vi "reporter2.vi"(1 "file path (dialog if empty)":path=path "C:/Users/Dimitris/Desktop/16_1_15.xls") -> (0 "output array 2":string[][](array[string]))   [LabVIEW 2012]
uses:
  <vilib>/Utility/file.llb/Write To Spreadsheet File (string).vi
  <vilib>/Utility/file.llb/Read From Spreadsheet File (DBL).vi
panel:
  out "output array 4":string[][](array[string])
  out "radiation_array 3":dbl[](array[numeric])
  out "radiation_array 2":dbl[](array[numeric])
  out "Panel7 acc":dbl[](array[numeric])
  out "Panel7 array":dbl[](array[numeric])
  out "Panel 6 acc":dbl[](array[numeric])
  out "Panel 6 array":dbl[](array[numeric])
  out "Panel 5 acc":dbl[](array[numeric])
  out "Panel 5 array":dbl[](array[numeric])
  out "Panel 4 acc":dbl[](array[numeric])
  out "Panel 4 array":dbl[](array[numeric])
  out "Panel 3 acc":dbl[](array[numeric])
  out "Panel 3 wp":dbl[](array[numeric])
  out "Panel 3 array":dbl[](array[numeric])
  out "Panel 2 wp":dbl[](array[numeric])
  out "Panel 1 wp":dbl[](array[numeric])
  out "Panel 1 acc":dbl[](array[numeric])
  out "Panel 1 array":dbl[](array[numeric])
  out "Panel 2_acc":dbl[](array[numeric])
  out "Panel 2 array":dbl[](array[numeric])
  out "radiation_array":dbl[](array[numeric])
  out "output array 3":string[][](array[string])
  out "output array":string[](array[string])
  out "8 13":i32
  out "rad_ 20":dbl
  out "panel1_20":dbl
  out "panel2_ 20":dbl
  out "panel3_20":dbl
  out "panel4_ 20":dbl
  out "panel5_20":dbl
  out "panel6_20":dbl
  out "panel7_20":dbl
  out "rad1_20":dbl
  out "rad2_20":dbl
  out "8 12":i32
  out "rad_ 19":dbl
  out "panel1_19":dbl
  out "panel2_ 19":dbl
  out "panel3_19":dbl
  out "panel4_ 19":dbl
  out "panel5_19":dbl
  out "panel6_19":dbl
  out "panel7_19":dbl
  out "rad1_19":dbl
  out "rad2_19":dbl
  out "8 11":i32
  out "rad_ 18":dbl
  out "panel1_18":dbl
  out "panel2_ 18":dbl
  out "panel3_18":dbl
  out "panel4_ 18":dbl
  out "panel5_18":dbl
  out "panel6_18":dbl
  out "panel7_18":dbl
  out "rad1_18":dbl
  out "rad2_18":dbl
  out "8 10":i32
  out "rad_ 17":dbl
  out "panel1_17":dbl
  out "panel2_ 17":dbl
  out "panel3_17":dbl
  out "panel4_ 17":dbl
  out "panel5_17":dbl
  out "panel6_17":dbl
  out "panel7_17":dbl
  out "rad1_17":dbl
  out "rad2_17":dbl
  out "8 9":i32
  out "rad_ 16":dbl
  out "panel1_16":dbl
  out "panel2_ 16":dbl
  out "panel3_16":dbl
  out "panel4_ 16":dbl
  out "panel5_16":dbl
  out "panel6_16":dbl
  out "panel7_16":dbl
  out "rad1_16":dbl
  out "rad2_16":dbl
  out "8 8":i32
  out "rad_ 15":dbl
  out "panel1_15":dbl
  out "panel2_ 15":dbl
  out "panel3_15":dbl
  out "panel4_ 15":dbl
  out "panel5_15":dbl
  out "panel6_15":dbl
  out "panel7_15":dbl
  out "rad1_15":dbl
  out "rad2_15":dbl
  out "8 7":i32
  out "rad_ 14":dbl
  out "panel1_14":dbl
  out "panel2_ 14":dbl
  out "panel3_14":dbl
  out "panel4_ 14":dbl
  out "panel5_14":dbl
  out "panel6_14":dbl
  out "panel7_14":dbl
  out "rad1_14":dbl
  out "rad2_14":dbl
  out "8 6":i32
  out "rad_ 13":dbl
  out "panel1_13":dbl
  out "panel2_ 13":dbl
  out "panel3_13":dbl
  out "panel4_ 13":dbl
  out "panel5_13":dbl
  out "panel6_13":dbl
  out "panel7_13":dbl
  out "rad1_13":dbl
  out "rad2_13":dbl
  out "8 5":i32
  out "rad_ 12":dbl
  out "panel1_12":dbl
  out "panel2_ 12":dbl
  out "panel3_12":dbl
  out "panel4_ 12":dbl
  out "panel5_12":dbl
  out "panel6_12":dbl
  out "panel7_12":dbl
  out "rad1_12":dbl
  out "rad2_12":dbl
  out "8 4":i32
  out "rad_ 11":dbl
  out "panel1_11":dbl
  out "panel2_ 11":dbl
  out "panel3_11":dbl
  out "panel4_ 11":dbl
  out "panel5_11":dbl
  out "panel6_11":dbl
  out "panel7_11":dbl
  out "rad1_11":dbl
  out "rad2_11":dbl
  out "8 3":i32
  out "rad_10":dbl
  out "panel1_10":dbl
  out "panel2_10":dbl
  out "panel3_10":dbl
  out "panel4_10":dbl
  out "panel5_10":dbl
  out "panel6_10":dbl
  out "panel7_10":dbl
  out "rad1_10":dbl
  out "rad2_10":dbl
  out "8 2":i32
  out "rad_9":dbl
  out "panel1_9":dbl
  out "panel2_9":dbl
  out "panel3_9":dbl
  out "panel4_9":dbl
  out "panel5_9":dbl
  out "panel6_9":dbl
  out "panel7_9":dbl
  out "rad1_9":dbl
  out "rad2_9":dbl
  out "8":i32
  out "rad_8":dbl
  out "panel1_8":dbl
  out "panel2_8":dbl
  out "panel3_8":dbl
  out "panel4_8":dbl
  out "panel5_8":dbl
  out "panel6_8":dbl
  out "panel7_8":dbl
  out "rad1_8":dbl
  out "rad2_8":dbl
  out "rad2_7":dbl
  out "rad1_7":dbl
  out "panel7_7":dbl
  out "panel6_7":dbl
  out "panel5_7":dbl
  out "all rows":dbl[][](array[numeric]) format="%0.3f"
  in  "column headers":string[](array[string])=["07am-08am", "08am-09am", "09am-10am", "10am-11am", "11am-12am", "12am-13pm", "13pm-14pm", "14pm-15pm", "15pm-16pm", "16pm-17pm", "17pm-18pm", "18pm-19pm", "19pm-20pm", "20pm-21pm"]
  out "appended array":dbl[][](array[numeric]) format="%#.3g"
  out "panel4_7":dbl
  out "panel3_7":dbl
  out "panel2_7":dbl
  out "panel1_7":dbl
  out "rad_7":dbl
  out "7":i32
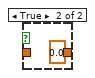
[diagram p2: hidden frame]
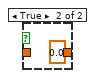
[diagram p3: hidden frame]
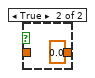
[diagram p4: hidden frame]
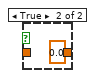
[diagram p5: hidden frame]
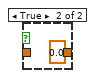
[diagram p6: hidden frame]
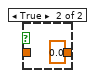
[diagram p7: hidden frame]
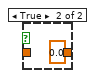
[diagram p8: hidden frame]
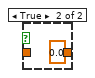
[diagram p9: hidden frame]
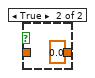
[diagram p10: hidden frame]
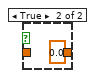
[diagram p11: hidden frame]
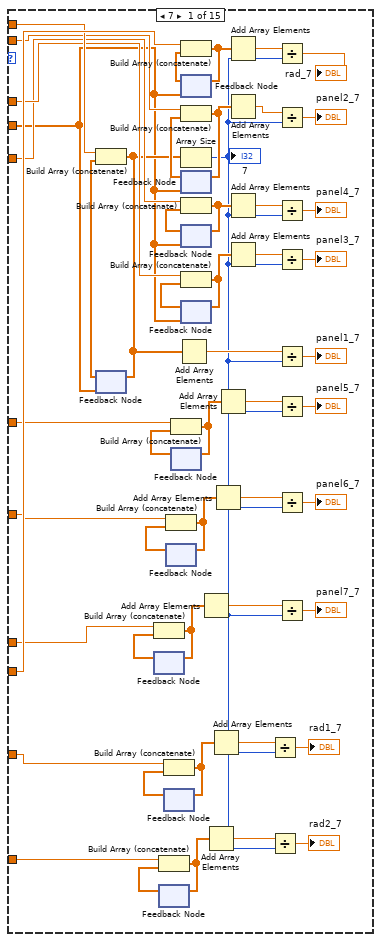
[diagram p12: hidden frame]
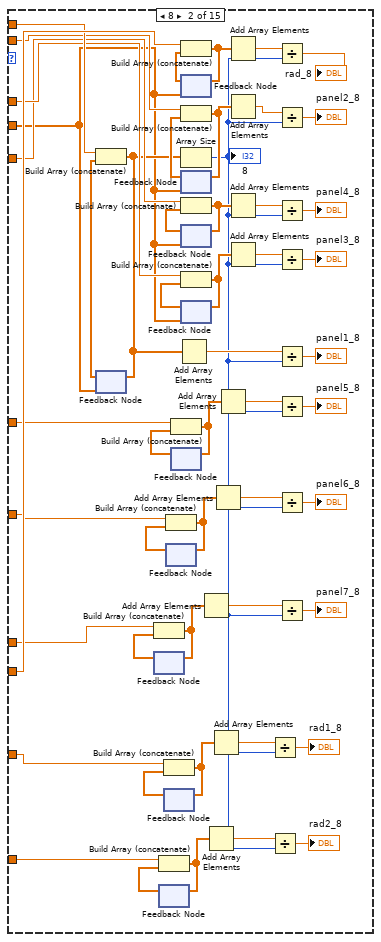
[diagram p13: hidden frame]
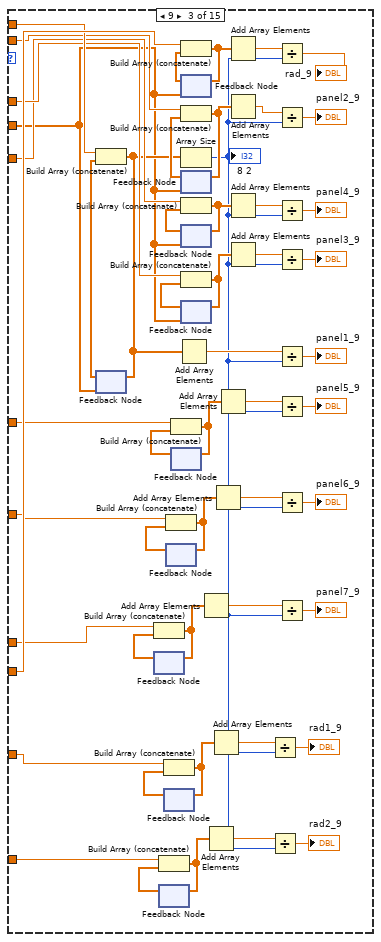
[diagram p14: hidden frame]
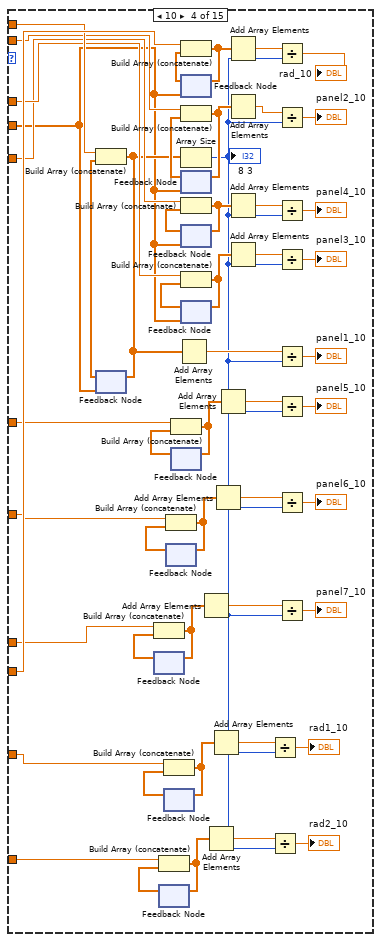
[diagram p15: hidden frame]
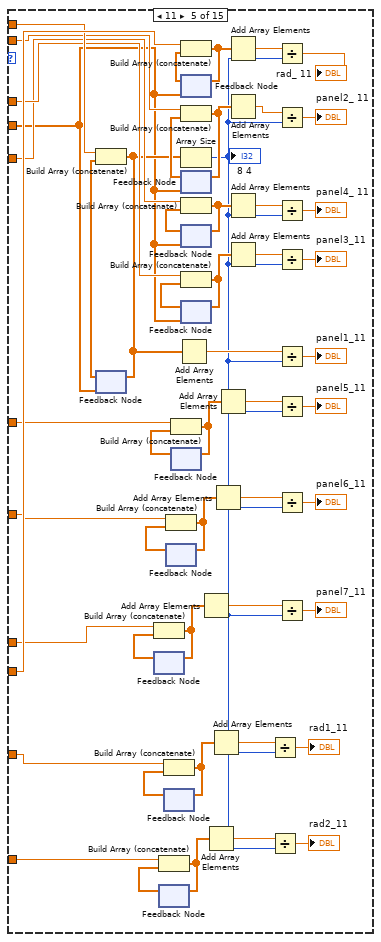
[diagram p16: hidden frame]
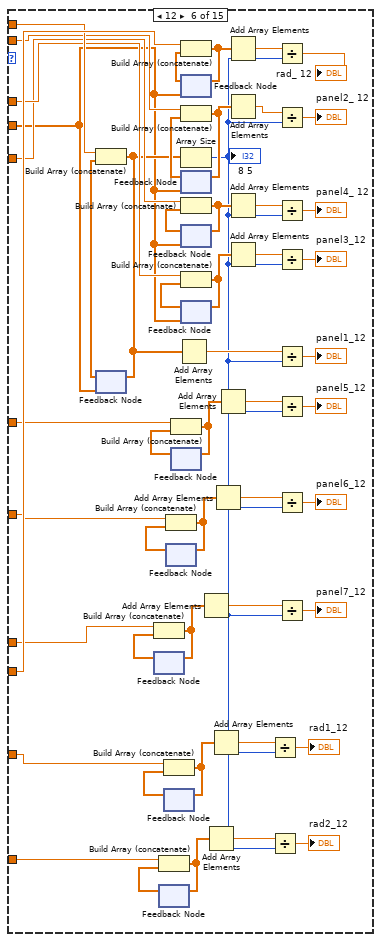
[diagram p17: hidden frame]
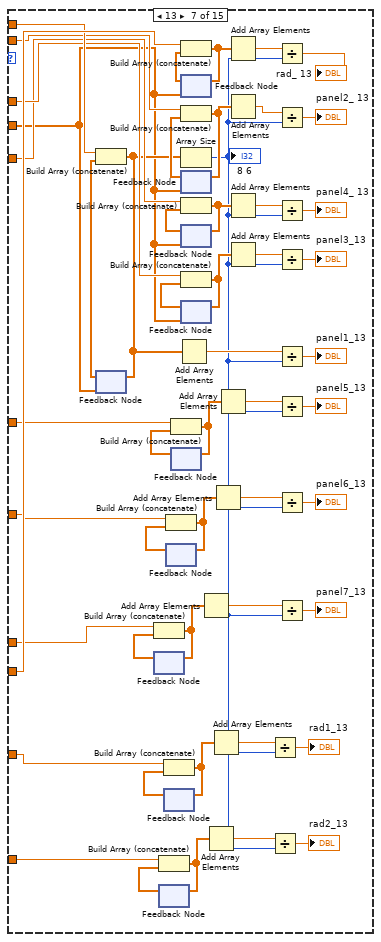
[diagram p18: hidden frame]
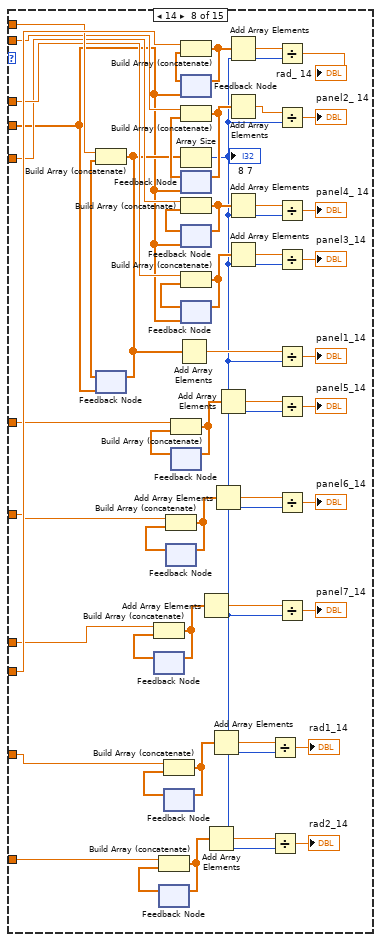
[diagram p19: hidden frame]
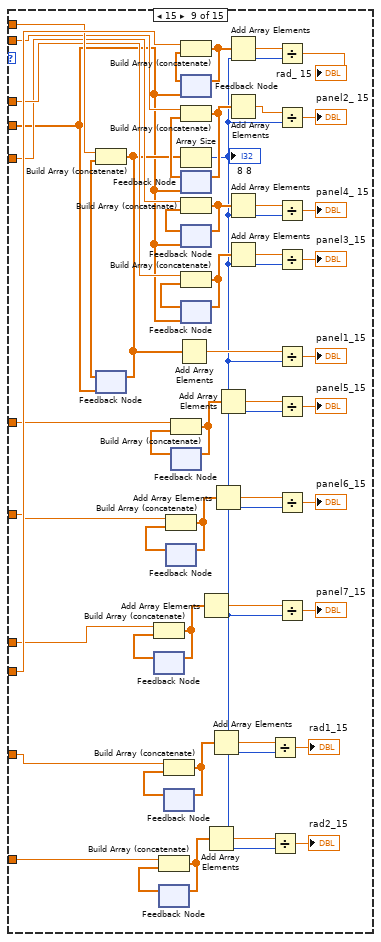
[diagram p20: hidden frame]
diagram:
  (unwired) FALSE ("use system decimal point (T)")
  w4 = string[] [" ", "Measured Wp- DSSC 1", "Measured Wp- DSSC 2", "Measured Wp- DSSC 3", "Measured Wp- Poly Si 1", "Measured Wp- Poly Si 2", "Measured Wp- Thin Film 1", "Measured Wp- Thin Film 2", "Accumulative Energy DSSC 1", "Accumulative Energy DSSC 2", "Accumulative Energy DSSC 3", "Accumulative Energy PolySi 1", "Accumulative Energy PolySi 2", "Accumulative Energy Film  1", "Accumulative Energy Film  2", "Wh/Wp  DSSC 1", "Wh/Wp  DSSC 2", "Wh/Wp  DSSC 3      ", "Wh/Wp  Poly Si  1    ", "Wh/Wp  Poly Si  2     ", "Wh/Wp  Thin Film 1", " Wh/Wp  Thin Film 2      ", "Radiation 1          ", "Radiation 2          ", "Radiation 3      ", " Radiation (meteo)          "] ("row headers")
  w22 = i16 3 ("precision (6)")
  w28 = "-" ("new element/subarray")
  n1 = property on="Panel 1 array" class="Arr (strict)" props=["Value"]() -> ()  [unwired: 2 in, 3 out]
  n2 = property on="Panel 1 wp" class="Arr (strict)" props=["Value"]() -> ()  [unwired: 2 in, 3 out]
  n3 = property on="Panel 1 acc" class="Arr (strict)" props=["Value"]() -> ()  [unwired: 2 in, 3 out]
  n4 = flat-sequence {
    tunnel: [w878] -> w9
    tunnel: [w895] -> w61
    tunnel: [w896] -> w69
    tunnel: [w893] -> w44
    tunnel: [w925] -> w58
    tunnel: [w927] -> w68
    tunnel: [w924] -> w41
    tunnel: [w956] -> w55
    tunnel: [w958] -> w67
    tunnel: [w955] -> w38
    tunnel: [w987] -> w52
    tunnel: [w989] -> w66
    tunnel: [w973] -> w10
    tunnel: [w1006] -> _
    tunnel: [w1005] -> _
    tunnel: [w1004] -> _
    tunnel: [w1037] -> _
    tunnel: [w1036] -> _
    tunnel: [w1035] -> _
    tunnel: [w1068] -> _
    tunnel: [w1067] -> _
    tunnel: [w1066] -> _
    tunnel: [w1127] -> w2
    frame #0 {
      n5 = call-poly <vilib>:"Read From Spreadsheet File.vi"("file path (dialog if empty)"="file path (dialog if empty)") -> ("all rows"=w71:dbl[][])  [unwired: 6 in, 4 out]
      "all rows" <- w71
      n6 = for {
        tunnel: w71 -> [w116] mode=indexing
        tunnel: dbl[] [] -> [w108]
        n7 = Index Array(array=w116, index #1=0 ("index"), index #2=1 ("index"), index #3=2 ("index"), index #4=3 ("index"), index #5=4 ("index"), index #6=5 ("index"), index #7=6 ("index"), index #8=7 ("index"), index #9=8 ("index"), index #10=9 ("index"), index #11=10 ("index")) -> (element #1=w110:dbl, element #2=w106:dbl, element #3=w98:dbl, element #4=w104:dbl, element #5=w99:dbl, element #6=w102:dbl, element #7=w91:dbl, element #8=w89:dbl, element #9=w87:dbl, element #10=w85:dbl, element #11=w82:dbl)
        n8 = Less Than 0?(x=w85) -> (x < 0?=w86:bool)
        n9 = Less Than 0?(x=w82) -> (x < 0?=w83:bool)
        n10 = Less Than 0?(x=w87) -> (x < 0?=w88:bool)
        n11 = Less Than 0?(x=w91) -> (x < 0?=w92:bool)
        n12 = Less Than 0?(x=w89) -> (x < 0?=w90:bool)
        n13 = case shown="False" w86 {
          tunnel: w85 -> [w119 _]
          tunnel: [w119 0.0] -> w84
          frame False {
          }
          frame True {
          }
        }
        n14 = Less Than 0?(x=w106) -> (x < 0?=w107:bool)
        n15 = Less Than 0?(x=w104) -> (x < 0?=w105:bool)
        n16 = Less Than 0?(x=w102) -> (x < 0?=w103:bool)
        n17 = Less Than 0?(x=w99) -> (x < 0?=w101:bool)
        n18 = Less Than 0?(x=w98) -> (x < 0?=w100:bool)
        n19 = case shown="False" w83 {
          tunnel: w82 -> [w117 _]
          tunnel: [w117 0.0] -> w81
          frame False {
          }
          frame True {
          }
        }
        n20 = case shown="False" w88 {
          tunnel: w87 -> [w121 _]
          tunnel: [w121 0.0] -> w76
          frame False {
          }
          frame True {
          }
        }
        n21 = case shown="False" w92 {
          tunnel: w91 -> [w125 _]
          tunnel: [w125 0.0] -> w74
          frame False {
          }
          frame True {
          }
        }
        n22 = case shown="False" w90 {
          tunnel: w89 -> [w123 _]
          tunnel: [w123 0.0] -> w73
          frame False {
          }
          frame True {
          }
        }
        n23 = case shown="False" w107 {
          tunnel: w106 -> [w135 _]
          tunnel: [w135 0.0] -> w80
          frame False {
          }
          frame True {
          }
        }
        n24 = case shown="False" w105 {
          tunnel: w104 -> [w133 _]
          tunnel: [w133 0.0] -> w79
          frame False {
          }
          frame True {
          }
        }
        n25 = case shown="False" w103 {
          tunnel: w102 -> [w131 _]
          tunnel: [w131 0.0] -> w78
          frame False {
          }
          frame True {
          }
        }
        n26 = case shown="False" w101 {
          tunnel: w99 -> [w129 _]
          tunnel: [w129 0.0] -> w77
          frame False {
          }
          frame True {
          }
        }
        n27 = case shown="False" w100 {
          tunnel: w98 -> [w127 _]
          tunnel: [w127 0.0] -> w75
          frame False {
          }
          frame True {
          }
        }
        n28 = case shown="20" w110 {
          tunnel: w76 -> [w188 w240 w292 w344 w396 w448 w500 w552 w604 w656 w708 w760 w812 w864 _]
          tunnel: w80 -> [w184 w236 w288 w340 w392 w444 w496 w548 w600 w652 w704 w756 w808 w860 _]
          tunnel: w79 -> [w183 w235 w287 w339 w391 w443 w495 w547 w599 w651 w703 w755 w807 w859 _]
          tunnel: w78 -> [w181 w233 w285 w337 w389 w441 w493 w545 w597 w649 w701 w753 w805 w857 _]
          tunnel: w77 -> [w179 w231 w283 w335 w387 w439 w491 w543 w595 w647 w699 w751 w803 w855 _]
          tunnel: w108 -> [w163 w215 w267 w319 w371 w423 w475 w527 w579 w631 w683 w735 w787 w839 _]
          tunnel: w75 -> [w158 w210 w262 w314 w366 w418 w470 w522 w574 w626 w678 w730 w782 w834 _]
          tunnel: w74 -> [w149 w201 w253 w305 w357 w409 w461 w513 w565 w617 w669 w721 w773 w825 _]
          tunnel: w73 -> [w148 w200 w252 w304 w356 w408 w460 w512 w564 w616 w668 w720 w772 w824 _]
          tunnel: w84 -> [w138 w190 w242 w294 w346 w398 w450 w502 w554 w606 w658 w710 w762 w814 _]
          tunnel: w81 -> [w137 w189 w241 w293 w345 w397 w449 w501 w553 w605 w657 w709 w761 w813 _]
          frame 7 {
            n29 = feedback #1(w163) -> (w186:dbl[])
            n30 = Build Array (concatenate)(w184, w186) -> (w167:dbl[])
            n31 = feedback-in #1(w167) -> ()
            n32 = feedback #2() -> (w153:dbl[])  [unwired: 1 in]
            n33 = Build Array (concatenate)(w148, w153) -> (w150:dbl[])
            n34 = feedback-in #2(w150) -> ()
            n35 = feedback #3() -> (w143:dbl[])  [unwired: 1 in]
            n36 = Build Array (concatenate)(w137, w143) -> (w140:dbl[])
            n37 = feedback-in #3(w140) -> ()
            n38 = feedback #4() -> (w147:dbl[])  [unwired: 1 in]
            n39 = Build Array (concatenate)(w138, w147) -> (w144:dbl[])
            n40 = feedback-in #4(w144) -> ()
            n41 = feedback #5() -> (w157:dbl[])  [unwired: 1 in]
            n42 = Build Array (concatenate)(w149, w157) -> (w154:dbl[])
            n43 = feedback-in #5(w154) -> ()
            n44 = feedback #6() -> (w162:dbl[])  [unwired: 1 in]
            n45 = Build Array (concatenate)(w158, w162) -> (w159:dbl[])
            n46 = feedback-in #6(w159) -> ()
            n47 = Add Array Elements(numeric array=w167) -> (sum=w170:dbl)
            n48 = feedback #7(w163) -> (w187:dbl[])
            n49 = Build Array (concatenate)(w188, w187) -> (w168:dbl[])
            n50 = feedback-in #7(w168) -> ()
            n51 = Array Size(array=w167) -> (size(s)=w139:i32)
            "7" <- w139
            n52 = feedback #8(w163) -> (w185:dbl[])
            n53 = Build Array (concatenate)(w183, w185) -> (w166:dbl[])
            n54 = feedback-in #8(w166) -> ()
            n55 = feedback #9(w163) -> (w180:dbl[])
            n56 = Build Array (concatenate)(w179, w180) -> (w164:dbl[])
            n57 = feedback-in #9(w164) -> ()
            n58 = feedback #10(w163) -> (w182:dbl[])
            n59 = Build Array (concatenate)(w181, w182) -> (w165:dbl[])
            n60 = feedback-in #10(w165) -> ()
            n61 = Add Array Elements(numeric array=w150) -> (sum=w151:dbl)
            n62 = Add Array Elements(numeric array=w140) -> (sum=w141:dbl)
            n63 = Add Array Elements(numeric array=w144) -> (sum=w145:dbl)
            n64 = Add Array Elements(numeric array=w154) -> (sum=w155:dbl)
            n65 = Add Array Elements(numeric array=w159) -> (sum=w160:dbl)
            n66 = Add Array Elements(numeric array=w168) -> (sum=w169:dbl)
            n67 = Add Array Elements(numeric array=w166) -> (sum=w172:dbl)
            n68 = Add Array Elements(numeric array=w164) -> (sum=w176:dbl)
            n69 = Add Array Elements(numeric array=w165) -> (sum=w174:dbl)
            n70 = Divide(x=w145, y=w139) -> (x/y=→"rad1_7":dbl)
            n71 = Divide(x=w141, y=w139) -> (x/y=→"rad2_7":dbl)
            n72 = Divide(x=w169, y=w139) -> (x/y=→"rad_7":dbl)
            n73 = Divide(x=w172, y=w139) -> (x/y=→"panel2_7":dbl)
            n74 = Divide(x=w176, y=w139) -> (x/y=→"panel4_7":dbl)
            n75 = Divide(x=w174, y=w139) -> (x/y=→"panel3_7":dbl)
            n76 = Divide(x=w170, y=w139) -> (x/y=→"panel1_7":dbl)
            n77 = Divide(x=w160, y=w139) -> (x/y=→"panel5_7":dbl)
            n78 = Divide(x=w155, y=w139) -> (x/y=→"panel6_7":dbl)
            n79 = Divide(x=w151, y=w139) -> (x/y=→"panel7_7":dbl)
          }
          frame 8 {
            n80 = feedback #11(w215) -> (w238:dbl[])
            n81 = Build Array (concatenate)(w236, w238) -> (w219:dbl[])
            n82 = feedback-in #11(w219) -> ()
            n83 = feedback #12() -> (w205:dbl[])  [unwired: 1 in]
            n84 = Build Array (concatenate)(w200, w205) -> (w202:dbl[])
            n85 = feedback-in #12(w202) -> ()
            n86 = feedback #13() -> (w195:dbl[])  [unwired: 1 in]
            n87 = Build Array (concatenate)(w189, w195) -> (w192:dbl[])
            n88 = feedback-in #13(w192) -> ()
            n89 = feedback #14() -> (w199:dbl[])  [unwired: 1 in]
            n90 = Build Array (concatenate)(w190, w199) -> (w196:dbl[])
            n91 = feedback-in #14(w196) -> ()
            n92 = feedback #15() -> (w209:dbl[])  [unwired: 1 in]
            n93 = Build Array (concatenate)(w201, w209) -> (w206:dbl[])
            n94 = feedback-in #15(w206) -> ()
            n95 = feedback #16() -> (w214:dbl[])  [unwired: 1 in]
            n96 = Build Array (concatenate)(w210, w214) -> (w211:dbl[])
            n97 = feedback-in #16(w211) -> ()
            n98 = Add Array Elements(numeric array=w219) -> (sum=w222:dbl)
            n99 = feedback #17(w215) -> (w239:dbl[])
            n100 = Build Array (concatenate)(w240, w239) -> (w220:dbl[])
            n101 = feedback-in #17(w220) -> ()
            n102 = Array Size(array=w219) -> (size(s)=w191:i32)
            "8" <- w191
            n103 = feedback #18(w215) -> (w237:dbl[])
            n104 = Build Array (concatenate)(w235, w237) -> (w218:dbl[])
            n105 = feedback-in #18(w218) -> ()
            n106 = feedback #19(w215) -> (w232:dbl[])
            n107 = Build Array (concatenate)(w231, w232) -> (w216:dbl[])
            n108 = feedback-in #19(w216) -> ()
            n109 = feedback #20(w215) -> (w234:dbl[])
            n110 = Build Array (concatenate)(w233, w234) -> (w217:dbl[])
            n111 = feedback-in #20(w217) -> ()
            n112 = Add Array Elements(numeric array=w202) -> (sum=w203:dbl)
            n113 = Add Array Elements(numeric array=w192) -> (sum=w193:dbl)
            n114 = Add Array Elements(numeric array=w196) -> (sum=w197:dbl)
            n115 = Add Array Elements(numeric array=w206) -> (sum=w207:dbl)
            n116 = Add Array Elements(numeric array=w211) -> (sum=w212:dbl)
            n117 = Add Array Elements(numeric array=w220) -> (sum=w221:dbl)
            n118 = Add Array Elements(numeric array=w218) -> (sum=w224:dbl)
            n119 = Add Array Elements(numeric array=w216) -> (sum=w228:dbl)
            n120 = Add Array Elements(numeric array=w217) -> (sum=w226:dbl)
            n121 = Divide(x=w197, y=w191) -> (x/y=→"rad1_8":dbl)
            n122 = Divide(x=w193, y=w191) -> (x/y=→"rad2_8":dbl)
            n123 = Divide(x=w221, y=w191) -> (x/y=→"rad_8":dbl)
            n124 = Divide(x=w224, y=w191) -> (x/y=→"panel2_8":dbl)
            n125 = Divide(x=w228, y=w191) -> (x/y=→"panel4_8":dbl)
            n126 = Divide(x=w226, y=w191) -> (x/y=→"panel3_8":dbl)
            n127 = Divide(x=w222, y=w191) -> (x/y=→"panel1_8":dbl)
            n128 = Divide(x=w212, y=w191) -> (x/y=→"panel5_8":dbl)
            n129 = Divide(x=w207, y=w191) -> (x/y=→"panel6_8":dbl)
            n130 = Divide(x=w203, y=w191) -> (x/y=→"panel7_8":dbl)
          }
          frame 9 {
            n131 = feedback #21(w267) -> (w290:dbl[])
            n132 = Build Array (concatenate)(w288, w290) -> (w271:dbl[])
            n133 = feedback-in #21(w271) -> ()
            n134 = feedback #22() -> (w257:dbl[])  [unwired: 1 in]
            n135 = Build Array (concatenate)(w252, w257) -> (w254:dbl[])
            n136 = feedback-in #22(w254) -> ()
            n137 = feedback #23() -> (w247:dbl[])  [unwired: 1 in]
            n138 = Build Array (concatenate)(w241, w247) -> (w244:dbl[])
            n139 = feedback-in #23(w244) -> ()
            n140 = feedback #24() -> (w251:dbl[])  [unwired: 1 in]
            n141 = Build Array (concatenate)(w242, w251) -> (w248:dbl[])
            n142 = feedback-in #24(w248) -> ()
            n143 = feedback #25() -> (w261:dbl[])  [unwired: 1 in]
            n144 = Build Array (concatenate)(w253, w261) -> (w258:dbl[])
            n145 = feedback-in #25(w258) -> ()
            n146 = feedback #26() -> (w266:dbl[])  [unwired: 1 in]
            n147 = Build Array (concatenate)(w262, w266) -> (w263:dbl[])
            n148 = feedback-in #26(w263) -> ()
            n149 = Add Array Elements(numeric array=w271) -> (sum=w274:dbl)
            n150 = feedback #27(w267) -> (w291:dbl[])
            n151 = Build Array (concatenate)(w292, w291) -> (w272:dbl[])
            n152 = feedback-in #27(w272) -> ()
            n153 = Array Size(array=w271) -> (size(s)=w243:i32)
            "8 2" <- w243
            n154 = feedback #28(w267) -> (w289:dbl[])
            n155 = Build Array (concatenate)(w287, w289) -> (w270:dbl[])
            n156 = feedback-in #28(w270) -> ()
            n157 = feedback #29(w267) -> (w284:dbl[])
            n158 = Build Array (concatenate)(w283, w284) -> (w268:dbl[])
            n159 = feedback-in #29(w268) -> ()
            n160 = feedback #30(w267) -> (w286:dbl[])
            n161 = Build Array (concatenate)(w285, w286) -> (w269:dbl[])
            n162 = feedback-in #30(w269) -> ()
            n163 = Add Array Elements(numeric array=w254) -> (sum=w255:dbl)
            n164 = Add Array Elements(numeric array=w244) -> (sum=w245:dbl)
            n165 = Add Array Elements(numeric array=w248) -> (sum=w249:dbl)
            n166 = Add Array Elements(numeric array=w258) -> (sum=w259:dbl)
            n167 = Add Array Elements(numeric array=w263) -> (sum=w264:dbl)
            n168 = Add Array Elements(numeric array=w272) -> (sum=w273:dbl)
            n169 = Add Array Elements(numeric array=w270) -> (sum=w276:dbl)
            n170 = Add Array Elements(numeric array=w268) -> (sum=w280:dbl)
            n171 = Add Array Elements(numeric array=w269) -> (sum=w278:dbl)
            n172 = Divide(x=w249, y=w243) -> (x/y=→"rad1_9":dbl)
            n173 = Divide(x=w245, y=w243) -> (x/y=→"rad2_9":dbl)
            n174 = Divide(x=w273, y=w243) -> (x/y=→"rad_9":dbl)
            n175 = Divide(x=w276, y=w243) -> (x/y=→"panel2_9":dbl)
            n176 = Divide(x=w280, y=w243) -> (x/y=→"panel4_9":dbl)
            n177 = Divide(x=w278, y=w243) -> (x/y=→"panel3_9":dbl)
            n178 = Divide(x=w274, y=w243) -> (x/y=→"panel1_9":dbl)
            n179 = Divide(x=w264, y=w243) -> (x/y=→"panel5_9":dbl)
            n180 = Divide(x=w259, y=w243) -> (x/y=→"panel6_9":dbl)
            n181 = Divide(x=w255, y=w243) -> (x/y=→"panel7_9":dbl)
          }
          frame 10 {
            n182 = feedback #31(w319) -> (w342:dbl[])
            n183 = Build Array (concatenate)(w340, w342) -> (w323:dbl[])
            n184 = feedback-in #31(w323) -> ()
            n185 = feedback #32() -> (w309:dbl[])  [unwired: 1 in]
            n186 = Build Array (concatenate)(w304, w309) -> (w306:dbl[])
            n187 = feedback-in #32(w306) -> ()
            n188 = feedback #33() -> (w299:dbl[])  [unwired: 1 in]
            n189 = Build Array (concatenate)(w293, w299) -> (w296:dbl[])
            n190 = feedback-in #33(w296) -> ()
            n191 = feedback #34() -> (w303:dbl[])  [unwired: 1 in]
            n192 = Build Array (concatenate)(w294, w303) -> (w300:dbl[])
            n193 = feedback-in #34(w300) -> ()
            n194 = feedback #35() -> (w313:dbl[])  [unwired: 1 in]
            n195 = Build Array (concatenate)(w305, w313) -> (w310:dbl[])
            n196 = feedback-in #35(w310) -> ()
            n197 = feedback #36() -> (w318:dbl[])  [unwired: 1 in]
            n198 = Build Array (concatenate)(w314, w318) -> (w315:dbl[])
            n199 = feedback-in #36(w315) -> ()
            n200 = Add Array Elements(numeric array=w323) -> (sum=w326:dbl)
            n201 = feedback #37(w319) -> (w343:dbl[])
            n202 = Build Array (concatenate)(w344, w343) -> (w324:dbl[])
            n203 = feedback-in #37(w324) -> ()
            n204 = Array Size(array=w323) -> (size(s)=w295:i32)
            "8 3" <- w295
            n205 = feedback #38(w319) -> (w341:dbl[])
            n206 = Build Array (concatenate)(w339, w341) -> (w322:dbl[])
            n207 = feedback-in #38(w322) -> ()
            n208 = feedback #39(w319) -> (w336:dbl[])
            n209 = Build Array (concatenate)(w335, w336) -> (w320:dbl[])
            n210 = feedback-in #39(w320) -> ()
            n211 = feedback #40(w319) -> (w338:dbl[])
            n212 = Build Array (concatenate)(w337, w338) -> (w321:dbl[])
            n213 = feedback-in #40(w321) -> ()
            n214 = Add Array Elements(numeric array=w306) -> (sum=w307:dbl)
            n215 = Add Array Elements(numeric array=w296) -> (sum=w297:dbl)
            n216 = Add Array Elements(numeric array=w300) -> (sum=w301:dbl)
            n217 = Add Array Elements(numeric array=w310) -> (sum=w311:dbl)
            n218 = Add Array Elements(numeric array=w315) -> (sum=w316:dbl)
            n219 = Add Array Elements(numeric array=w324) -> (sum=w325:dbl)
            n220 = Add Array Elements(numeric array=w322) -> (sum=w328:dbl)
            n221 = Add Array Elements(numeric array=w320) -> (sum=w332:dbl)
            n222 = Add Array Elements(numeric array=w321) -> (sum=w330:dbl)
            n223 = Divide(x=w301, y=w295) -> (x/y=→"rad1_10":dbl)
            n224 = Divide(x=w297, y=w295) -> (x/y=→"rad2_10":dbl)
            n225 = Divide(x=w325, y=w295) -> (x/y=→"rad_10":dbl)
            n226 = Divide(x=w328, y=w295) -> (x/y=→"panel2_10":dbl)
            n227 = Divide(x=w332, y=w295) -> (x/y=→"panel4_10":dbl)
            n228 = Divide(x=w330, y=w295) -> (x/y=→"panel3_10":dbl)
            n229 = Divide(x=w326, y=w295) -> (x/y=→"panel1_10":dbl)
            n230 = Divide(x=w316, y=w295) -> (x/y=→"panel5_10":dbl)
            n231 = Divide(x=w311, y=w295) -> (x/y=→"panel6_10":dbl)
            n232 = Divide(x=w307, y=w295) -> (x/y=→"panel7_10":dbl)
          }
          frame 11 {
            n233 = feedback #41(w371) -> (w394:dbl[])
            n234 = Build Array (concatenate)(w392, w394) -> (w375:dbl[])
            n235 = feedback-in #41(w375) -> ()
            n236 = feedback #42() -> (w361:dbl[])  [unwired: 1 in]
            n237 = Build Array (concatenate)(w356, w361) -> (w358:dbl[])
            n238 = feedback-in #42(w358) -> ()
            n239 = feedback #43() -> (w351:dbl[])  [unwired: 1 in]
            n240 = Build Array (concatenate)(w345, w351) -> (w348:dbl[])
            n241 = feedback-in #43(w348) -> ()
            n242 = feedback #44() -> (w355:dbl[])  [unwired: 1 in]
            n243 = Build Array (concatenate)(w346, w355) -> (w352:dbl[])
            n244 = feedback-in #44(w352) -> ()
            n245 = feedback #45() -> (w365:dbl[])  [unwired: 1 in]
            n246 = Build Array (concatenate)(w357, w365) -> (w362:dbl[])
            n247 = feedback-in #45(w362) -> ()
            n248 = feedback #46() -> (w370:dbl[])  [unwired: 1 in]
            n249 = Build Array (concatenate)(w366, w370) -> (w367:dbl[])
            n250 = feedback-in #46(w367) -> ()
            n251 = Add Array Elements(numeric array=w375) -> (sum=w378:dbl)
            n252 = feedback #47(w371) -> (w395:dbl[])
            n253 = Build Array (concatenate)(w396, w395) -> (w376:dbl[])
            n254 = feedback-in #47(w376) -> ()
            n255 = Array Size(array=w375) -> (size(s)=w347:i32)
            "8 4" <- w347
            n256 = feedback #48(w371) -> (w393:dbl[])
            n257 = Build Array (concatenate)(w391, w393) -> (w374:dbl[])
            n258 = feedback-in #48(w374) -> ()
            n259 = feedback #49(w371) -> (w388:dbl[])
            n260 = Build Array (concatenate)(w387, w388) -> (w372:dbl[])
            n261 = feedback-in #49(w372) -> ()
            n262 = feedback #50(w371) -> (w390:dbl[])
            n263 = Build Array (concatenate)(w389, w390) -> (w373:dbl[])
            n264 = feedback-in #50(w373) -> ()
            n265 = Add Array Elements(numeric array=w358) -> (sum=w359:dbl)
            n266 = Add Array Elements(numeric array=w348) -> (sum=w349:dbl)
            n267 = Add Array Elements(numeric array=w352) -> (sum=w353:dbl)
            n268 = Add Array Elements(numeric array=w362) -> (sum=w363:dbl)
            n269 = Add Array Elements(numeric array=w367) -> (sum=w368:dbl)
            n270 = Add Array Elements(numeric array=w376) -> (sum=w377:dbl)
            n271 = Add Array Elements(numeric array=w374) -> (sum=w380:dbl)
            n272 = Add Array Elements(numeric array=w372) -> (sum=w384:dbl)
            n273 = Add Array Elements(numeric array=w373) -> (sum=w382:dbl)
            n274 = Divide(x=w353, y=w347) -> (x/y=→"rad1_11":dbl)
            n275 = Divide(x=w349, y=w347) -> (x/y=→"rad2_11":dbl)
            n276 = Divide(x=w377, y=w347) -> (x/y=→"rad_ 11":dbl)
            n277 = Divide(x=w380, y=w347) -> (x/y=→"panel2_ 11":dbl)
            n278 = Divide(x=w384, y=w347) -> (x/y=→"panel4_ 11":dbl)
            n279 = Divide(x=w382, y=w347) -> (x/y=→"panel3_11":dbl)
            n280 = Divide(x=w378, y=w347) -> (x/y=→"panel1_11":dbl)
            n281 = Divide(x=w368, y=w347) -> (x/y=→"panel5_11":dbl)
            n282 = Divide(x=w363, y=w347) -> (x/y=→"panel6_11":dbl)
            n283 = Divide(x=w359, y=w347) -> (x/y=→"panel7_11":dbl)
          }
          frame 12 {
            n284 = feedback #51(w423) -> (w446:dbl[])
            n285 = Build Array (concatenate)(w444, w446) -> (w427:dbl[])
            n286 = feedback-in #51(w427) -> ()
            n287 = feedback #52() -> (w413:dbl[])  [unwired: 1 in]
            n288 = Build Array (concatenate)(w408, w413) -> (w410:dbl[])
            n289 = feedback-in #52(w410) -> ()
            n290 = feedback #53() -> (w403:dbl[])  [unwired: 1 in]
            n291 = Build Array (concatenate)(w397, w403) -> (w400:dbl[])
            n292 = feedback-in #53(w400) -> ()
            n293 = feedback #54() -> (w407:dbl[])  [unwired: 1 in]
            n294 = Build Array (concatenate)(w398, w407) -> (w404:dbl[])
            n295 = feedback-in #54(w404) -> ()
            n296 = feedback #55() -> (w417:dbl[])  [unwired: 1 in]
            n297 = Build Array (concatenate)(w409, w417) -> (w414:dbl[])
            n298 = feedback-in #55(w414) -> ()
            n299 = feedback #56() -> (w422:dbl[])  [unwired: 1 in]
            n300 = Build Array (concatenate)(w418, w422) -> (w419:dbl[])
            n301 = feedback-in #56(w419) -> ()
            n302 = Add Array Elements(numeric array=w427) -> (sum=w430:dbl)
            n303 = feedback #57(w423) -> (w447:dbl[])
            n304 = Build Array (concatenate)(w448, w447) -> (w428:dbl[])
            n305 = feedback-in #57(w428) -> ()
            n306 = Array Size(array=w427) -> (size(s)=w399:i32)
            "8 5" <- w399
            n307 = feedback #58(w423) -> (w445:dbl[])
            n308 = Build Array (concatenate)(w443, w445) -> (w426:dbl[])
            n309 = feedback-in #58(w426) -> ()
            n310 = feedback #59(w423) -> (w440:dbl[])
            n311 = Build Array (concatenate)(w439, w440) -> (w424:dbl[])
            n312 = feedback-in #59(w424) -> ()
            n313 = feedback #60(w423) -> (w442:dbl[])
            n314 = Build Array (concatenate)(w441, w442) -> (w425:dbl[])
            n315 = feedback-in #60(w425) -> ()
            n316 = Add Array Elements(numeric array=w410) -> (sum=w411:dbl)
            n317 = Add Array Elements(numeric array=w400) -> (sum=w401:dbl)
            n318 = Add Array Elements(numeric array=w404) -> (sum=w405:dbl)
            n319 = Add Array Elements(numeric array=w414) -> (sum=w415:dbl)
            n320 = Add Array Elements(numeric array=w419) -> (sum=w420:dbl)
            n321 = Add Array Elements(numeric array=w428) -> (sum=w429:dbl)
            n322 = Add Array Elements(numeric array=w426) -> (sum=w432:dbl)
            n323 = Add Array Elements(numeric array=w424) -> (sum=w436:dbl)
            n324 = Add Array Elements(numeric array=w425) -> (sum=w434:dbl)
            n325 = Divide(x=w405, y=w399) -> (x/y=→"rad1_12":dbl)
            n326 = Divide(x=w401, y=w399) -> (x/y=→"rad2_12":dbl)
            n327 = Divide(x=w429, y=w399) -> (x/y=→"rad_ 12":dbl)
            n328 = Divide(x=w432, y=w399) -> (x/y=→"panel2_ 12":dbl)
            n329 = Divide(x=w436, y=w399) -> (x/y=→"panel4_ 12":dbl)
            n330 = Divide(x=w434, y=w399) -> (x/y=→"panel3_12":dbl)
            n331 = Divide(x=w430, y=w399) -> (x/y=→"panel1_12":dbl)
            n332 = Divide(x=w420, y=w399) -> (x/y=→"panel5_12":dbl)
            n333 = Divide(x=w415, y=w399) -> (x/y=→"panel6_12":dbl)
            n334 = Divide(x=w411, y=w399) -> (x/y=→"panel7_12":dbl)
          }
          frame 13 {
            n335 = feedback #61(w475) -> (w498:dbl[])
            n336 = Build Array (concatenate)(w496, w498) -> (w479:dbl[])
            n337 = feedback-in #61(w479) -> ()
            n338 = feedback #62() -> (w465:dbl[])  [unwired: 1 in]
            n339 = Build Array (concatenate)(w460, w465) -> (w462:dbl[])
            n340 = feedback-in #62(w462) -> ()
            n341 = feedback #63() -> (w455:dbl[])  [unwired: 1 in]
            n342 = Build Array (concatenate)(w449, w455) -> (w452:dbl[])
            n343 = feedback-in #63(w452) -> ()
            n344 = feedback #64() -> (w459:dbl[])  [unwired: 1 in]
            n345 = Build Array (concatenate)(w450, w459) -> (w456:dbl[])
            n346 = feedback-in #64(w456) -> ()
            n347 = feedback #65() -> (w469:dbl[])  [unwired: 1 in]
            n348 = Build Array (concatenate)(w461, w469) -> (w466:dbl[])
            n349 = feedback-in #65(w466) -> ()
            n350 = feedback #66() -> (w474:dbl[])  [unwired: 1 in]
            n351 = Build Array (concatenate)(w470, w474) -> (w471:dbl[])
            n352 = feedback-in #66(w471) -> ()
            n353 = Add Array Elements(numeric array=w479) -> (sum=w482:dbl)
            n354 = feedback #67(w475) -> (w499:dbl[])
            n355 = Build Array (concatenate)(w500, w499) -> (w480:dbl[])
            n356 = feedback-in #67(w480) -> ()
            n357 = Array Size(array=w479) -> (size(s)=w451:i32)
            "8 6" <- w451
            n358 = feedback #68(w475) -> (w497:dbl[])
            n359 = Build Array (concatenate)(w495, w497) -> (w478:dbl[])
            n360 = feedback-in #68(w478) -> ()
            n361 = feedback #69(w475) -> (w492:dbl[])
            n362 = Build Array (concatenate)(w491, w492) -> (w476:dbl[])
            n363 = feedback-in #69(w476) -> ()
            n364 = feedback #70(w475) -> (w494:dbl[])
            n365 = Build Array (concatenate)(w493, w494) -> (w477:dbl[])
            n366 = feedback-in #70(w477) -> ()
            n367 = Add Array Elements(numeric array=w462) -> (sum=w463:dbl)
            n368 = Add Array Elements(numeric array=w452) -> (sum=w453:dbl)
            n369 = Add Array Elements(numeric array=w456) -> (sum=w457:dbl)
            n370 = Add Array Elements(numeric array=w466) -> (sum=w467:dbl)
            n371 = Add Array Elements(numeric array=w471) -> (sum=w472:dbl)
            n372 = Add Array Elements(numeric array=w480) -> (sum=w481:dbl)
            n373 = Add Array Elements(numeric array=w478) -> (sum=w484:dbl)
            n374 = Add Array Elements(numeric array=w476) -> (sum=w488:dbl)
            n375 = Add Array Elements(numeric array=w477) -> (sum=w486:dbl)
            n376 = Divide(x=w457, y=w451) -> (x/y=→"rad1_13":dbl)
            n377 = Divide(x=w453, y=w451) -> (x/y=→"rad2_13":dbl)
            n378 = Divide(x=w481, y=w451) -> (x/y=→"rad_ 13":dbl)
            n379 = Divide(x=w484, y=w451) -> (x/y=→"panel2_ 13":dbl)
            n380 = Divide(x=w488, y=w451) -> (x/y=→"panel4_ 13":dbl)
            n381 = Divide(x=w486, y=w451) -> (x/y=→"panel3_13":dbl)
            n382 = Divide(x=w482, y=w451) -> (x/y=→"panel1_13":dbl)
            n383 = Divide(x=w472, y=w451) -> (x/y=→"panel5_13":dbl)
            n384 = Divide(x=w467, y=w451) -> (x/y=→"panel6_13":dbl)
            n385 = Divide(x=w463, y=w451) -> (x/y=→"panel7_13":dbl)
          }
          frame 14 {
            n386 = feedback #71(w527) -> (w550:dbl[])
            n387 = Build Array (concatenate)(w548, w550) -> (w531:dbl[])
            n388 = feedback-in #71(w531) -> ()
            n389 = feedback #72() -> (w517:dbl[])  [unwired: 1 in]
            n390 = Build Array (concatenate)(w512, w517) -> (w514:dbl[])
            n391 = feedback-in #72(w514) -> ()
            n392 = feedback #73() -> (w507:dbl[])  [unwired: 1 in]
            n393 = Build Array (concatenate)(w501, w507) -> (w504:dbl[])
            n394 = feedback-in #73(w504) -> ()
            n395 = feedback #74() -> (w511:dbl[])  [unwired: 1 in]
            n396 = Build Array (concatenate)(w502, w511) -> (w508:dbl[])
            n397 = feedback-in #74(w508) -> ()
            n398 = feedback #75() -> (w521:dbl[])  [unwired: 1 in]
            n399 = Build Array (concatenate)(w513, w521) -> (w518:dbl[])
            n400 = feedback-in #75(w518) -> ()
            n401 = feedback #76() -> (w526:dbl[])  [unwired: 1 in]
            n402 = Build Array (concatenate)(w522, w526) -> (w523:dbl[])
            n403 = feedback-in #76(w523) -> ()
            n404 = Add Array Elements(numeric array=w531) -> (sum=w534:dbl)
            n405 = feedback #77(w527) -> (w551:dbl[])
            n406 = Build Array (concatenate)(w552, w551) -> (w532:dbl[])
            n407 = feedback-in #77(w532) -> ()
            n408 = Array Size(array=w531) -> (size(s)=w503:i32)
            "8 7" <- w503
            n409 = feedback #78(w527) -> (w549:dbl[])
            n410 = Build Array (concatenate)(w547, w549) -> (w530:dbl[])
            n411 = feedback-in #78(w530) -> ()
            n412 = feedback #79(w527) -> (w544:dbl[])
            n413 = Build Array (concatenate)(w543, w544) -> (w528:dbl[])
            n414 = feedback-in #79(w528) -> ()
            n415 = feedback #80(w527) -> (w546:dbl[])
            n416 = Build Array (concatenate)(w545, w546) -> (w529:dbl[])
            n417 = feedback-in #80(w529) -> ()
            n418 = Add Array Elements(numeric array=w514) -> (sum=w515:dbl)
            n419 = Add Array Elements(numeric array=w504) -> (sum=w505:dbl)
            n420 = Add Array Elements(numeric array=w508) -> (sum=w509:dbl)
            n421 = Add Array Elements(numeric array=w518) -> (sum=w519:dbl)
            n422 = Add Array Elements(numeric array=w523) -> (sum=w524:dbl)
            n423 = Add Array Elements(numeric array=w532) -> (sum=w533:dbl)
            n424 = Add Array Elements(numeric array=w530) -> (sum=w536:dbl)
            n425 = Add Array Elements(numeric array=w528) -> (sum=w540:dbl)
            n426 = Add Array Elements(numeric array=w529) -> (sum=w538:dbl)
            n427 = Divide(x=w509, y=w503) -> (x/y=→"rad1_14":dbl)
            n428 = Divide(x=w505, y=w503) -> (x/y=→"rad2_14":dbl)
            n429 = Divide(x=w533, y=w503) -> (x/y=→"rad_ 14":dbl)
            n430 = Divide(x=w536, y=w503) -> (x/y=→"panel2_ 14":dbl)
            n431 = Divide(x=w540, y=w503) -> (x/y=→"panel4_ 14":dbl)
            n432 = Divide(x=w538, y=w503) -> (x/y=→"panel3_14":dbl)
            n433 = Divide(x=w534, y=w503) -> (x/y=→"panel1_14":dbl)
            n434 = Divide(x=w524, y=w503) -> (x/y=→"panel5_14":dbl)
            n435 = Divide(x=w519, y=w503) -> (x/y=→"panel6_14":dbl)
            n436 = Divide(x=w515, y=w503) -> (x/y=→"panel7_14":dbl)
          }
          frame 15 {
            n437 = feedback #81(w579) -> (w602:dbl[])
            n438 = Build Array (concatenate)(w600, w602) -> (w583:dbl[])
            n439 = feedback-in #81(w583) -> ()
            n440 = feedback #82() -> (w569:dbl[])  [unwired: 1 in]
            n441 = Build Array (concatenate)(w564, w569) -> (w566:dbl[])
            n442 = feedback-in #82(w566) -> ()
            n443 = feedback #83() -> (w559:dbl[])  [unwired: 1 in]
            n444 = Build Array (concatenate)(w553, w559) -> (w556:dbl[])
            n445 = feedback-in #83(w556) -> ()
            n446 = feedback #84() -> (w563:dbl[])  [unwired: 1 in]
            n447 = Build Array (concatenate)(w554, w563) -> (w560:dbl[])
            n448 = feedback-in #84(w560) -> ()
            n449 = feedback #85() -> (w573:dbl[])  [unwired: 1 in]
            n450 = Build Array (concatenate)(w565, w573) -> (w570:dbl[])
            n451 = feedback-in #85(w570) -> ()
            n452 = feedback #86() -> (w578:dbl[])  [unwired: 1 in]
            n453 = Build Array (concatenate)(w574, w578) -> (w575:dbl[])
            n454 = feedback-in #86(w575) -> ()
            n455 = Add Array Elements(numeric array=w583) -> (sum=w586:dbl)
            n456 = feedback #87(w579) -> (w603:dbl[])
            n457 = Build Array (concatenate)(w604, w603) -> (w584:dbl[])
            n458 = feedback-in #87(w584) -> ()
            n459 = Array Size(array=w583) -> (size(s)=w555:i32)
            "8 8" <- w555
            n460 = feedback #88(w579) -> (w601:dbl[])
            n461 = Build Array (concatenate)(w599, w601) -> (w582:dbl[])
            n462 = feedback-in #88(w582) -> ()
            n463 = feedback #89(w579) -> (w596:dbl[])
            n464 = Build Array (concatenate)(w595, w596) -> (w580:dbl[])
            n465 = feedback-in #89(w580) -> ()
            n466 = feedback #90(w579) -> (w598:dbl[])
            n467 = Build Array (concatenate)(w597, w598) -> (w581:dbl[])
            n468 = feedback-in #90(w581) -> ()
            n469 = Add Array Elements(numeric array=w566) -> (sum=w567:dbl)
            n470 = Add Array Elements(numeric array=w556) -> (sum=w557:dbl)
            n471 = Add Array Elements(numeric array=w560) -> (sum=w561:dbl)
            n472 = Add Array Elements(numeric array=w570) -> (sum=w571:dbl)
            n473 = Add Array Elements(numeric array=w575) -> (sum=w576:dbl)
            n474 = Add Array Elements(numeric array=w584) -> (sum=w585:dbl)
            n475 = Add Array Elements(numeric array=w582) -> (sum=w588:dbl)
            n476 = Add Array Elements(numeric array=w580) -> (sum=w592:dbl)
            n477 = Add Array Elements(numeric array=w581) -> (sum=w590:dbl)
            n478 = Divide(x=w561, y=w555) -> (x/y=→"rad1_15":dbl)
            n479 = Divide(x=w557, y=w555) -> (x/y=→"rad2_15":dbl)
            n480 = Divide(x=w585, y=w555) -> (x/y=→"rad_ 15":dbl)
            n481 = Divide(x=w588, y=w555) -> (x/y=→"panel2_ 15":dbl)
            n482 = Divide(x=w592, y=w555) -> (x/y=→"panel4_ 15":dbl)
            n483 = Divide(x=w590, y=w555) -> (x/y=→"panel3_15":dbl)
            n484 = Divide(x=w586, y=w555) -> (x/y=→"panel1_15":dbl)
            n485 = Divide(x=w576, y=w555) -> (x/y=→"panel5_15":dbl)
            n486 = Divide(x=w571, y=w555) -> (x/y=→"panel6_15":dbl)
            n487 = Divide(x=w567, y=w555) -> (x/y=→"panel7_15":dbl)
          }
          frame 16 {
            n488 = feedback #91(w631) -> (w654:dbl[])
            n489 = Build Array (concatenate)(w652, w654) -> (w635:dbl[])
            n490 = feedback-in #91(w635) -> ()
            n491 = feedback #92() -> (w621:dbl[])  [unwired: 1 in]
            n492 = Build Array (concatenate)(w616, w621) -> (w618:dbl[])
            n493 = feedback-in #92(w618) -> ()
            n494 = feedback #93() -> (w611:dbl[])  [unwired: 1 in]
            n495 = Build Array (concatenate)(w605, w611) -> (w608:dbl[])
            n496 = feedback-in #93(w608) -> ()
            n497 = feedback #94() -> (w615:dbl[])  [unwired: 1 in]
            n498 = Build Array (concatenate)(w606, w615) -> (w612:dbl[])
            n499 = feedback-in #94(w612) -> ()
            n500 = feedback #95() -> (w625:dbl[])  [unwired: 1 in]
            n501 = Build Array (concatenate)(w617, w625) -> (w622:dbl[])
            n502 = feedback-in #95(w622) -> ()
            n503 = feedback #96() -> (w630:dbl[])  [unwired: 1 in]
            n504 = Build Array (concatenate)(w626, w630) -> (w627:dbl[])
            n505 = feedback-in #96(w627) -> ()
            n506 = Add Array Elements(numeric array=w635) -> (sum=w638:dbl)
            n507 = feedback #97(w631) -> (w655:dbl[])
            n508 = Build Array (concatenate)(w656, w655) -> (w636:dbl[])
            n509 = feedback-in #97(w636) -> ()
            n510 = Array Size(array=w635) -> (size(s)=w607:i32)
            "8 9" <- w607
            n511 = feedback #98(w631) -> (w653:dbl[])
            n512 = Build Array (concatenate)(w651, w653) -> (w634:dbl[])
            n513 = feedback-in #98(w634) -> ()
            n514 = feedback #99(w631) -> (w648:dbl[])
            n515 = Build Array (concatenate)(w647, w648) -> (w632:dbl[])
            n516 = feedback-in #99(w632) -> ()
            n517 = feedback #100(w631) -> (w650:dbl[])
            n518 = Build Array (concatenate)(w649, w650) -> (w633:dbl[])
            n519 = feedback-in #100(w633) -> ()
            n520 = Add Array Elements(numeric array=w618) -> (sum=w619:dbl)
            n521 = Add Array Elements(numeric array=w608) -> (sum=w609:dbl)
            n522 = Add Array Elements(numeric array=w612) -> (sum=w613:dbl)
            n523 = Add Array Elements(numeric array=w622) -> (sum=w623:dbl)
            n524 = Add Array Elements(numeric array=w627) -> (sum=w628:dbl)
            n525 = Add Array Elements(numeric array=w636) -> (sum=w637:dbl)
            n526 = Add Array Elements(numeric array=w634) -> (sum=w640:dbl)
            n527 = Add Array Elements(numeric array=w632) -> (sum=w644:dbl)
            n528 = Add Array Elements(numeric array=w633) -> (sum=w642:dbl)
            n529 = Divide(x=w613, y=w607) -> (x/y=→"rad1_16":dbl)
            n530 = Divide(x=w609, y=w607) -> (x/y=→"rad2_16":dbl)
            n531 = Divide(x=w637, y=w607) -> (x/y=→"rad_ 16":dbl)
            n532 = Divide(x=w640, y=w607) -> (x/y=→"panel2_ 16":dbl)
            n533 = Divide(x=w644, y=w607) -> (x/y=→"panel4_ 16":dbl)
            n534 = Divide(x=w642, y=w607) -> (x/y=→"panel3_16":dbl)
            n535 = Divide(x=w638, y=w607) -> (x/y=→"panel1_16":dbl)
            n536 = Divide(x=w628, y=w607) -> (x/y=→"panel5_16":dbl)
            n537 = Divide(x=w623, y=w607) -> (x/y=→"panel6_16":dbl)
            n538 = Divide(x=w619, y=w607) -> (x/y=→"panel7_16":dbl)
          }
          frame 17 {
            n539 = feedback #101(w683) -> (w706:dbl[])
            n540 = Build Array (concatenate)(w704, w706) -> (w687:dbl[])
            n541 = feedback-in #101(w687) -> ()
            n542 = feedback #102() -> (w673:dbl[])  [unwired: 1 in]
            n543 = Build Array (concatenate)(w668, w673) -> (w670:dbl[])
            n544 = feedback-in #102(w670) -> ()
            n545 = feedback #103() -> (w663:dbl[])  [unwired: 1 in]
            n546 = Build Array (concatenate)(w657, w663) -> (w660:dbl[])
            n547 = feedback-in #103(w660) -> ()
            n548 = feedback #104() -> (w667:dbl[])  [unwired: 1 in]
            n549 = Build Array (concatenate)(w658, w667) -> (w664:dbl[])
            n550 = feedback-in #104(w664) -> ()
            n551 = feedback #105() -> (w677:dbl[])  [unwired: 1 in]
            n552 = Build Array (concatenate)(w669, w677) -> (w674:dbl[])
            n553 = feedback-in #105(w674) -> ()
            n554 = feedback #106() -> (w682:dbl[])  [unwired: 1 in]
            n555 = Build Array (concatenate)(w678, w682) -> (w679:dbl[])
            n556 = feedback-in #106(w679) -> ()
            n557 = Add Array Elements(numeric array=w687) -> (sum=w690:dbl)
            n558 = feedback #107(w683) -> (w707:dbl[])
            n559 = Build Array (concatenate)(w708, w707) -> (w688:dbl[])
            n560 = feedback-in #107(w688) -> ()
            n561 = Array Size(array=w687) -> (size(s)=w659:i32)
            "8 10" <- w659
            n562 = feedback #108(w683) -> (w705:dbl[])
            n563 = Build Array (concatenate)(w703, w705) -> (w686:dbl[])
            n564 = feedback-in #108(w686) -> ()
            n565 = feedback #109(w683) -> (w700:dbl[])
            n566 = Build Array (concatenate)(w699, w700) -> (w684:dbl[])
            n567 = feedback-in #109(w684) -> ()
            n568 = feedback #110(w683) -> (w702:dbl[])
            n569 = Build Array (concatenate)(w701, w702) -> (w685:dbl[])
            n570 = feedback-in #110(w685) -> ()
            n571 = Add Array Elements(numeric array=w670) -> (sum=w671:dbl)
            n572 = Add Array Elements(numeric array=w660) -> (sum=w661:dbl)
            n573 = Add Array Elements(numeric array=w664) -> (sum=w665:dbl)
            n574 = Add Array Elements(numeric array=w674) -> (sum=w675:dbl)
            n575 = Add Array Elements(numeric array=w679) -> (sum=w680:dbl)
            n576 = Add Array Elements(numeric array=w688) -> (sum=w689:dbl)
            n577 = Add Array Elements(numeric array=w686) -> (sum=w692:dbl)
            n578 = Add Array Elements(numeric array=w684) -> (sum=w696:dbl)
            n579 = Add Array Elements(numeric array=w685) -> (sum=w694:dbl)
            n580 = Divide(x=w665, y=w659) -> (x/y=→"rad1_17":dbl)
            n581 = Divide(x=w661, y=w659) -> (x/y=→"rad2_17":dbl)
            n582 = Divide(x=w689, y=w659) -> (x/y=→"rad_ 17":dbl)
            n583 = Divide(x=w692, y=w659) -> (x/y=→"panel2_ 17":dbl)
            n584 = Divide(x=w696, y=w659) -> (x/y=→"panel4_ 17":dbl)
            n585 = Divide(x=w694, y=w659) -> (x/y=→"panel3_17":dbl)
            n586 = Divide(x=w690, y=w659) -> (x/y=→"panel1_17":dbl)
            n587 = Divide(x=w680, y=w659) -> (x/y=→"panel5_17":dbl)
            n588 = Divide(x=w675, y=w659) -> (x/y=→"panel6_17":dbl)
            n589 = Divide(x=w671, y=w659) -> (x/y=→"panel7_17":dbl)
          }
          frame 18 {
            n590 = feedback #111(w735) -> (w758:dbl[])
            n591 = Build Array (concatenate)(w756, w758) -> (w739:dbl[])
            n592 = feedback-in #111(w739) -> ()
            n593 = feedback #112() -> (w725:dbl[])  [unwired: 1 in]
            n594 = Build Array (concatenate)(w720, w725) -> (w722:dbl[])
            n595 = feedback-in #112(w722) -> ()
            n596 = feedback #113() -> (w715:dbl[])  [unwired: 1 in]
            n597 = Build Array (concatenate)(w709, w715) -> (w712:dbl[])
            n598 = feedback-in #113(w712) -> ()
            n599 = feedback #114() -> (w719:dbl[])  [unwired: 1 in]
            n600 = Build Array (concatenate)(w710, w719) -> (w716:dbl[])
            n601 = feedback-in #114(w716) -> ()
            n602 = feedback #115() -> (w729:dbl[])  [unwired: 1 in]
            n603 = Build Array (concatenate)(w721, w729) -> (w726:dbl[])
            n604 = feedback-in #115(w726) -> ()
            n605 = feedback #116() -> (w734:dbl[])  [unwired: 1 in]
            n606 = Build Array (concatenate)(w730, w734) -> (w731:dbl[])
            n607 = feedback-in #116(w731) -> ()
            n608 = Add Array Elements(numeric array=w739) -> (sum=w742:dbl)
            n609 = feedback #117(w735) -> (w759:dbl[])
            n610 = Build Array (concatenate)(w760, w759) -> (w740:dbl[])
            n611 = feedback-in #117(w740) -> ()
            n612 = Array Size(array=w739) -> (size(s)=w711:i32)
            "8 11" <- w711
            n613 = feedback #118(w735) -> (w757:dbl[])
            n614 = Build Array (concatenate)(w755, w757) -> (w738:dbl[])
            n615 = feedback-in #118(w738) -> ()
            n616 = feedback #119(w735) -> (w752:dbl[])
            n617 = Build Array (concatenate)(w751, w752) -> (w736:dbl[])
            n618 = feedback-in #119(w736) -> ()
            n619 = feedback #120(w735) -> (w754:dbl[])
            n620 = Build Array (concatenate)(w753, w754) -> (w737:dbl[])
            n621 = feedback-in #120(w737) -> ()
            n622 = Add Array Elements(numeric array=w722) -> (sum=w723:dbl)
            n623 = Add Array Elements(numeric array=w712) -> (sum=w713:dbl)
            n624 = Add Array Elements(numeric array=w716) -> (sum=w717:dbl)
            n625 = Add Array Elements(numeric array=w726) -> (sum=w727:dbl)
            n626 = Add Array Elements(numeric array=w731) -> (sum=w732:dbl)
            n627 = Add Array Elements(numeric array=w740) -> (sum=w741:dbl)
            n628 = Add Array Elements(numeric array=w738) -> (sum=w744:dbl)
            n629 = Add Array Elements(numeric array=w736) -> (sum=w748:dbl)
            n630 = Add Array Elements(numeric array=w737) -> (sum=w746:dbl)
            n631 = Divide(x=w717, y=w711) -> (x/y=→"rad1_18":dbl)
            n632 = Divide(x=w713, y=w711) -> (x/y=→"rad2_18":dbl)
            n633 = Divide(x=w741, y=w711) -> (x/y=→"rad_ 18":dbl)
            n634 = Divide(x=w744, y=w711) -> (x/y=→"panel2_ 18":dbl)
            n635 = Divide(x=w748, y=w711) -> (x/y=→"panel4_ 18":dbl)
            n636 = Divide(x=w746, y=w711) -> (x/y=→"panel3_18":dbl)
            n637 = Divide(x=w742, y=w711) -> (x/y=→"panel1_18":dbl)
            n638 = Divide(x=w732, y=w711) -> (x/y=→"panel5_18":dbl)
            n639 = Divide(x=w727, y=w711) -> (x/y=→"panel6_18":dbl)
            n640 = Divide(x=w723, y=w711) -> (x/y=→"panel7_18":dbl)
          }
          frame 19 {
            n641 = feedback #121(w787) -> (w810:dbl[])
            n642 = Build Array (concatenate)(w808, w810) -> (w791:dbl[])
            n643 = feedback-in #121(w791) -> ()
            n644 = feedback #122() -> (w777:dbl[])  [unwired: 1 in]
            n645 = Build Array (concatenate)(w772, w777) -> (w774:dbl[])
            n646 = feedback-in #122(w774) -> ()
            n647 = feedback #123() -> (w767:dbl[])  [unwired: 1 in]
            n648 = Build Array (concatenate)(w761, w767) -> (w764:dbl[])
            n649 = feedback-in #123(w764) -> ()
            n650 = feedback #124() -> (w771:dbl[])  [unwired: 1 in]
            n651 = Build Array (concatenate)(w762, w771) -> (w768:dbl[])
            n652 = feedback-in #124(w768) -> ()
            n653 = feedback #125() -> (w781:dbl[])  [unwired: 1 in]
            n654 = Build Array (concatenate)(w773, w781) -> (w778:dbl[])
            n655 = feedback-in #125(w778) -> ()
            n656 = feedback #126() -> (w786:dbl[])  [unwired: 1 in]
            n657 = Build Array (concatenate)(w782, w786) -> (w783:dbl[])
            n658 = feedback-in #126(w783) -> ()
            n659 = Add Array Elements(numeric array=w791) -> (sum=w794:dbl)
            n660 = feedback #127(w787) -> (w811:dbl[])
            n661 = Build Array (concatenate)(w812, w811) -> (w792:dbl[])
            n662 = feedback-in #127(w792) -> ()
            n663 = Array Size(array=w791) -> (size(s)=w763:i32)
            "8 12" <- w763
            n664 = feedback #128(w787) -> (w809:dbl[])
            n665 = Build Array (concatenate)(w807, w809) -> (w790:dbl[])
            n666 = feedback-in #128(w790) -> ()
            n667 = feedback #129(w787) -> (w804:dbl[])
            n668 = Build Array (concatenate)(w803, w804) -> (w788:dbl[])
            n669 = feedback-in #129(w788) -> ()
            n670 = feedback #130(w787) -> (w806:dbl[])
            n671 = Build Array (concatenate)(w805, w806) -> (w789:dbl[])
            n672 = feedback-in #130(w789) -> ()
            n673 = Add Array Elements(numeric array=w774) -> (sum=w775:dbl)
            n674 = Add Array Elements(numeric array=w764) -> (sum=w765:dbl)
            n675 = Add Array Elements(numeric array=w768) -> (sum=w769:dbl)
            n676 = Add Array Elements(numeric array=w778) -> (sum=w779:dbl)
            n677 = Add Array Elements(numeric array=w783) -> (sum=w784:dbl)
            n678 = Add Array Elements(numeric array=w792) -> (sum=w793:dbl)
            n679 = Add Array Elements(numeric array=w790) -> (sum=w796:dbl)
            n680 = Add Array Elements(numeric array=w788) -> (sum=w800:dbl)
            n681 = Add Array Elements(numeric array=w789) -> (sum=w798:dbl)
            n682 = Divide(x=w769, y=w763) -> (x/y=→"rad1_19":dbl)
            n683 = Divide(x=w765, y=w763) -> (x/y=→"rad2_19":dbl)
            n684 = Divide(x=w793, y=w763) -> (x/y=→"rad_ 19":dbl)
            n685 = Divide(x=w796, y=w763) -> (x/y=→"panel2_ 19":dbl)
            n686 = Divide(x=w800, y=w763) -> (x/y=→"panel4_ 19":dbl)
            n687 = Divide(x=w798, y=w763) -> (x/y=→"panel3_19":dbl)
            n688 = Divide(x=w794, y=w763) -> (x/y=→"panel1_19":dbl)
            n689 = Divide(x=w784, y=w763) -> (x/y=→"panel5_19":dbl)
            n690 = Divide(x=w779, y=w763) -> (x/y=→"panel6_19":dbl)
            n691 = Divide(x=w775, y=w763) -> (x/y=→"panel7_19":dbl)
          }
          frame 20 {
            n692 = feedback #131(w839) -> (w862:dbl[])
            n693 = Build Array (concatenate)(w860, w862) -> (w843:dbl[])
            n694 = feedback-in #131(w843) -> ()
            n695 = feedback #132() -> (w829:dbl[])  [unwired: 1 in]
            n696 = Build Array (concatenate)(w824, w829) -> (w826:dbl[])
            n697 = feedback-in #132(w826) -> ()
            n698 = feedback #133() -> (w819:dbl[])  [unwired: 1 in]
            n699 = Build Array (concatenate)(w813, w819) -> (w816:dbl[])
            n700 = feedback-in #133(w816) -> ()
            n701 = feedback #134() -> (w823:dbl[])  [unwired: 1 in]
            n702 = Build Array (concatenate)(w814, w823) -> (w820:dbl[])
            n703 = feedback-in #134(w820) -> ()
            n704 = feedback #135() -> (w833:dbl[])  [unwired: 1 in]
            n705 = Build Array (concatenate)(w825, w833) -> (w830:dbl[])
            n706 = feedback-in #135(w830) -> ()
            n707 = feedback #136() -> (w838:dbl[])  [unwired: 1 in]
            n708 = Build Array (concatenate)(w834, w838) -> (w835:dbl[])
            n709 = feedback-in #136(w835) -> ()
            n710 = Add Array Elements(numeric array=w843) -> (sum=w846:dbl)
            n711 = feedback #137(w839) -> (w863:dbl[])
            n712 = Build Array (concatenate)(w864, w863) -> (w844:dbl[])
            n713 = feedback-in #137(w844) -> ()
            n714 = Array Size(array=w843) -> (size(s)=w815:i32)
            "8 13" <- w815
            n715 = feedback #138(w839) -> (w861:dbl[])
            n716 = Build Array (concatenate)(w859, w861) -> (w842:dbl[])
            n717 = feedback-in #138(w842) -> ()
            n718 = feedback #139(w839) -> (w856:dbl[])
            n719 = Build Array (concatenate)(w855, w856) -> (w840:dbl[])
            n720 = feedback-in #139(w840) -> ()
            n721 = feedback #140(w839) -> (w858:dbl[])
            n722 = Build Array (concatenate)(w857, w858) -> (w841:dbl[])
            n723 = feedback-in #140(w841) -> ()
            n724 = Add Array Elements(numeric array=w826) -> (sum=w827:dbl)
            n725 = Add Array Elements(numeric array=w816) -> (sum=w817:dbl)
            n726 = Add Array Elements(numeric array=w820) -> (sum=w821:dbl)
            n727 = Add Array Elements(numeric array=w830) -> (sum=w831:dbl)
            n728 = Add Array Elements(numeric array=w835) -> (sum=w836:dbl)
            n729 = Add Array Elements(numeric array=w844) -> (sum=w845:dbl)
            n730 = Add Array Elements(numeric array=w842) -> (sum=w848:dbl)
            n731 = Add Array Elements(numeric array=w840) -> (sum=w852:dbl)
            n732 = Add Array Elements(numeric array=w841) -> (sum=w850:dbl)
            n733 = Divide(x=w821, y=w815) -> (x/y=→"rad1_20":dbl)
            n734 = Divide(x=w817, y=w815) -> (x/y=→"rad2_20":dbl)
            n735 = Divide(x=w845, y=w815) -> (x/y=→"rad_ 20":dbl)
            n736 = Divide(x=w848, y=w815) -> (x/y=→"panel2_ 20":dbl)
            n737 = Divide(x=w852, y=w815) -> (x/y=→"panel4_ 20":dbl)
            n738 = Divide(x=w850, y=w815) -> (x/y=→"panel3_20":dbl)
            n739 = Divide(x=w846, y=w815) -> (x/y=→"panel1_20":dbl)
            n740 = Divide(x=w836, y=w815) -> (x/y=→"panel5_20":dbl)
            n741 = Divide(x=w831, y=w815) -> (x/y=→"panel6_20":dbl)
            n742 = Divide(x=w827, y=w815) -> (x/y=→"panel7_20":dbl)
          }
          frame 0, Default {
          }
        }
      }
    }
    frame #1 {
      # "radiation"
      n743 = property on="rad_7" class="DigNum (strict)"() -> ("Value"=w879:dbl)  [unwired: 2 in, 2 out]
      n744 = property on="rad_8" class="DigNum (strict)"() -> ("Value"=w877:dbl)  [unwired: 2 in, 2 out]
      n745 = property on="rad_9" class="DigNum (strict)"() -> ("Value"=w865:dbl)  [unwired: 2 in, 2 out]
      n746 = property on="rad_10" class="DigNum (strict)"() -> ("Value"=w866:dbl)  [unwired: 2 in, 2 out]
      n747 = property on="rad_ 11" class="DigNum (strict)"() -> ("Value"=w867:dbl)  [unwired: 2 in, 2 out]
      n748 = property on="rad_ 12" class="DigNum (strict)"() -> ("Value"=w868:dbl)  [unwired: 2 in, 2 out]
      n749 = property on="rad_ 13" class="DigNum (strict)"() -> ("Value"=w869:dbl)  [unwired: 2 in, 2 out]
      n750 = property on="rad_ 14" class="DigNum (strict)"() -> ("Value"=w870:dbl)  [unwired: 2 in, 2 out]
      n751 = property on="rad_ 15" class="DigNum (strict)"() -> ("Value"=w871:dbl)  [unwired: 2 in, 2 out]
      n752 = property on="rad_ 16" class="DigNum (strict)"() -> ("Value"=w872:dbl)  [unwired: 2 in, 2 out]
      n753 = property on="rad_ 17" class="DigNum (strict)"() -> ("Value"=w873:dbl)  [unwired: 2 in, 2 out]
      n754 = property on="rad_ 18" class="DigNum (strict)"() -> ("Value"=w874:dbl)  [unwired: 2 in, 2 out]
      n755 = property on="rad_ 19" class="DigNum (strict)"() -> ("Value"=w875:dbl)  [unwired: 2 in, 2 out]
      n756 = property on="rad_ 20" class="DigNum (strict)"() -> ("Value"=w876:dbl)  [unwired: 2 in, 2 out]
      n757 = Build Array(w879, w877, w865, w866, w867, w868, w869, w870, w871, w872, w873, w874, w875, w876) -> (w878:dbl[])
      "radiation_array" <- w878
    }
    frame #2 {
      # "Panel 1"
      n758 = property on="panel1_7" class="DigNum (strict)"() -> ("Value"=w910:dbl)  [unwired: 2 in, 2 out]
      n759 = property on="panel1_8" class="DigNum (strict)"() -> ("Value"=w880:dbl)  [unwired: 2 in, 2 out]
      n760 = property on="panel1_9" class="DigNum (strict)"() -> ("Value"=w881:dbl)  [unwired: 2 in, 2 out]
      n761 = property on="panel1_10" class="DigNum (strict)"() -> ("Value"=w882:dbl)  [unwired: 2 in, 2 out]
      n762 = property on="panel1_11" class="DigNum (strict)"() -> ("Value"=w883:dbl)  [unwired: 2 in, 2 out]
      n763 = property on="panel1_12" class="DigNum (strict)"() -> ("Value"=w884:dbl)  [unwired: 2 in, 2 out]
      n764 = property on="panel1_13" class="DigNum (strict)"() -> ("Value"=w885:dbl)  [unwired: 2 in, 2 out]
      n765 = property on="panel1_14" class="DigNum (strict)"() -> ("Value"=w886:dbl)  [unwired: 2 in, 2 out]
      n766 = property on="panel1_15" class="DigNum (strict)"() -> ("Value"=w887:dbl)  [unwired: 2 in, 2 out]
      n767 = property on="panel1_16" class="DigNum (strict)"() -> ("Value"=w888:dbl)  [unwired: 2 in, 2 out]
      n768 = property on="panel1_17" class="DigNum (strict)"() -> ("Value"=w889:dbl)  [unwired: 2 in, 2 out]
      n769 = property on="panel1_18" class="DigNum (strict)"() -> ("Value"=w890:dbl)  [unwired: 2 in, 2 out]
      n770 = property on="panel1_19" class="DigNum (strict)"() -> ("Value"=w891:dbl)  [unwired: 2 in, 2 out]
      n771 = property on="panel1_20" class="DigNum (strict)"() -> ("Value"=w892:dbl)  [unwired: 2 in, 2 out]
      n772 = Build Array(w910, w880, w881, w882, w883, w884, w886, w885, w887, w888, w889, w890, w891, w892) -> (w895:dbl[])
      "Panel 1 array" <- w895
      n773 = Add(x=w910, y=w880) -> (x+y=w909:dbl)
      n774 = Add(x=w909, y=w881) -> (x+y=w908:dbl)
      n775 = Add(x=w908, y=w882) -> (x+y=w907:dbl)
      n776 = Add(x=w907, y=w883) -> (x+y=w906:dbl)
      n777 = Add(x=w906, y=w884) -> (x+y=w905:dbl)
      n778 = Add(x=w905, y=w886) -> (x+y=w904:dbl)
      n779 = Add(x=w904, y=w885) -> (x+y=w903:dbl)
      n780 = Divide(x=w895, y=160) -> (x/y=w893:dbl[])
      "Panel 1 wp" <- w893
      n781 = Add(x=w903, y=w887) -> (x+y=w902:dbl)
      n782 = Add(x=w902, y=w888) -> (x+y=w901:dbl)
      n783 = Add(x=w901, y=w889) -> (x+y=w900:dbl)
      n784 = Add(x=w900, y=w890) -> (x+y=w899:dbl)
      n785 = Add(x=w899, y=w891) -> (x+y=w897:dbl)
      n786 = Add(x=w897, y=w892) -> (x+y=w898:dbl)
      n787 = Build Array(w910, w909, w908, w907, w906, w905, w904, w903, w902, w901, w900, w899, w897, w898) -> (w896:dbl[])
      "Panel 1 acc" <- w896
    }
    frame #3 {
      # "panel 2"
      n788 = property on="panel2_7" class="DigNum (strict)"() -> ("Value"=w941:dbl)  [unwired: 2 in, 2 out]
      n789 = property on="panel2_8" class="DigNum (strict)"() -> ("Value"=w923:dbl)  [unwired: 2 in, 2 out]
      n790 = property on="panel2_9" class="DigNum (strict)"() -> ("Value"=w922:dbl)  [unwired: 2 in, 2 out]
      n791 = property on="panel2_10" class="DigNum (strict)"() -> ("Value"=w921:dbl)  [unwired: 2 in, 2 out]
      n792 = property on="panel2_ 11" class="DigNum (strict)"() -> ("Value"=w920:dbl)  [unwired: 2 in, 2 out]
      n793 = property on="panel2_ 12" class="DigNum (strict)"() -> ("Value"=w919:dbl)  [unwired: 2 in, 2 out]
      n794 = property on="panel2_ 13" class="DigNum (strict)"() -> ("Value"=w918:dbl)  [unwired: 2 in, 2 out]
      n795 = property on="panel2_ 14" class="DigNum (strict)"() -> ("Value"=w917:dbl)  [unwired: 2 in, 2 out]
      n796 = property on="panel2_ 15" class="DigNum (strict)"() -> ("Value"=w916:dbl)  [unwired: 2 in, 2 out]
      n797 = property on="panel2_ 16" class="DigNum (strict)"() -> ("Value"=w915:dbl)  [unwired: 2 in, 2 out]
      n798 = property on="panel2_ 17" class="DigNum (strict)"() -> ("Value"=w914:dbl)  [unwired: 2 in, 2 out]
      n799 = property on="panel2_ 18" class="DigNum (strict)"() -> ("Value"=w913:dbl)  [unwired: 2 in, 2 out]
      n800 = property on="panel2_ 19" class="DigNum (strict)"() -> ("Value"=w912:dbl)  [unwired: 2 in, 2 out]
      n801 = property on="panel2_ 20" class="DigNum (strict)"() -> ("Value"=w911:dbl)  [unwired: 2 in, 2 out]
      n802 = Add(x=w941, y=w923) -> (x+y=w940:dbl)
      n803 = Build Array(w941, w923, w922, w921, w920, w919, w918, w917, w916, w915, w914, w913, w912, w911) -> (w925:dbl[])
      "Panel 2 array" <- w925
      n804 = Add(x=w940, y=w922) -> (x+y=w939:dbl)
      n805 = Add(x=w939, y=w921) -> (x+y=w938:dbl)
      n806 = Add(x=w938, y=w920) -> (x+y=w937:dbl)
      n807 = Add(x=w937, y=w919) -> (x+y=w936:dbl)
      n808 = Add(x=w936, y=w918) -> (x+y=w935:dbl)
      n809 = Add(x=w935, y=w917) -> (x+y=w934:dbl)
      n810 = Add(x=w934, y=w916) -> (x+y=w933:dbl)
      n811 = Add(x=w933, y=w915) -> (x+y=w932:dbl)
      n812 = Add(x=w932, y=w914) -> (x+y=w931:dbl)
      n813 = Add(x=w931, y=w913) -> (x+y=w930:dbl)
      n814 = Add(x=w930, y=w912) -> (x+y=w928:dbl)
      n815 = Divide(x=w925, y=74.5) -> (x/y=w924:dbl[])
      "Panel 2 wp" <- w924
      n816 = Add(x=w928, y=w911) -> (x+y=w929:dbl)
      n817 = Build Array(w941, w940, w939, w938, w937, w936, w935, w934, w933, w932, w931, w930, w928, w929) -> (w927:dbl[])
      "Panel 2_acc" <- w927
    }
    frame #4 {
      # "panel 3"
      n818 = property on="panel3_7" class="DigNum (strict)"() -> ("Value"=w972:dbl)  [unwired: 2 in, 2 out]
      n819 = property on="panel3_8" class="DigNum (strict)"() -> ("Value"=w942:dbl)  [unwired: 2 in, 2 out]
      n820 = property on="panel3_9" class="DigNum (strict)"() -> ("Value"=w943:dbl)  [unwired: 2 in, 2 out]
      n821 = property on="panel3_10" class="DigNum (strict)"() -> ("Value"=w944:dbl)  [unwired: 2 in, 2 out]
      n822 = property on="panel3_11" class="DigNum (strict)"() -> ("Value"=w945:dbl)  [unwired: 2 in, 2 out]
      n823 = property on="panel3_12" class="DigNum (strict)"() -> ("Value"=w946:dbl)  [unwired: 2 in, 2 out]
      n824 = property on="panel3_13" class="DigNum (strict)"() -> ("Value"=w947:dbl)  [unwired: 2 in, 2 out]
      n825 = property on="panel3_14" class="DigNum (strict)"() -> ("Value"=w948:dbl)  [unwired: 2 in, 2 out]
      n826 = property on="panel3_15" class="DigNum (strict)"() -> ("Value"=w949:dbl)  [unwired: 2 in, 2 out]
      n827 = property on="panel3_16" class="DigNum (strict)"() -> ("Value"=w950:dbl)  [unwired: 2 in, 2 out]
      n828 = property on="panel3_17" class="DigNum (strict)"() -> ("Value"=w951:dbl)  [unwired: 2 in, 2 out]
      n829 = property on="panel3_18" class="DigNum (strict)"() -> ("Value"=w952:dbl)  [unwired: 2 in, 2 out]
      n830 = property on="panel3_19" class="DigNum (strict)"() -> ("Value"=w953:dbl)  [unwired: 2 in, 2 out]
      n831 = property on="panel3_20" class="DigNum (strict)"() -> ("Value"=w954:dbl)  [unwired: 2 in, 2 out]
      n832 = Build Array(w972, w942, w943, w944, w945, w946, w947, w948, w949, w950, w951, w952, w953, w954) -> (w956:dbl[])
      "Panel 3 array" <- w956
      n833 = Add(x=w972, y=w942) -> (x+y=w971:dbl)
      n834 = Add(x=w971, y=w943) -> (x+y=w970:dbl)
      n835 = Add(x=w970, y=w944) -> (x+y=w969:dbl)
      n836 = Add(x=w969, y=w945) -> (x+y=w968:dbl)
      n837 = Add(x=w968, y=w946) -> (x+y=w967:dbl)
      n838 = Add(x=w967, y=w947) -> (x+y=w966:dbl)
      n839 = Add(x=w966, y=w948) -> (x+y=w965:dbl)
      n840 = Add(x=w965, y=w949) -> (x+y=w964:dbl)
      n841 = Divide(x=w956, y=18) -> (x/y=w955:dbl[])
      "Panel 3 wp" <- w955
      n842 = Add(x=w964, y=w950) -> (x+y=w963:dbl)
      n843 = Add(x=w963, y=w951) -> (x+y=w962:dbl)
      n844 = Add(x=w962, y=w952) -> (x+y=w961:dbl)
      n845 = Add(x=w961, y=w953) -> (x+y=w959:dbl)
      n846 = Add(x=w959, y=w954) -> (x+y=w960:dbl)
      n847 = Build Array(w972, w971, w970, w969, w968, w967, w966, w965, w964, w963, w962, w961, w959, w960) -> (w958:dbl[])
      "Panel 3 acc" <- w958
    }
    frame #5 {
      # "panel 4"
      n848 = property on="panel4_8" class="DigNum (strict)"() -> ("Value"=w974:dbl)  [unwired: 2 in, 2 out]
      n849 = property on="panel4_9" class="DigNum (strict)"() -> ("Value"=w975:dbl)  [unwired: 2 in, 2 out]
      n850 = property on="panel4_10" class="DigNum (strict)"() -> ("Value"=w976:dbl)  [unwired: 2 in, 2 out]
      n851 = property on="panel4_ 11" class="DigNum (strict)"() -> ("Value"=w977:dbl)  [unwired: 2 in, 2 out]
      n852 = property on="panel4_ 12" class="DigNum (strict)"() -> ("Value"=w978:dbl)  [unwired: 2 in, 2 out]
      n853 = property on="panel4_ 13" class="DigNum (strict)"() -> ("Value"=w979:dbl)  [unwired: 2 in, 2 out]
      n854 = property on="panel4_ 14" class="DigNum (strict)"() -> ("Value"=w980:dbl)  [unwired: 2 in, 2 out]
      n855 = property on="panel4_ 15" class="DigNum (strict)"() -> ("Value"=w981:dbl)  [unwired: 2 in, 2 out]
      n856 = property on="panel4_ 16" class="DigNum (strict)"() -> ("Value"=w982:dbl)  [unwired: 2 in, 2 out]
      n857 = property on="panel4_ 17" class="DigNum (strict)"() -> ("Value"=w983:dbl)  [unwired: 2 in, 2 out]
      n858 = property on="panel4_ 18" class="DigNum (strict)"() -> ("Value"=w984:dbl)  [unwired: 2 in, 2 out]
      n859 = property on="panel4_ 19" class="DigNum (strict)"() -> ("Value"=w985:dbl)  [unwired: 2 in, 2 out]
      n860 = property on="panel4_ 20" class="DigNum (strict)"() -> ("Value"=w986:dbl)  [unwired: 2 in, 2 out]
      n861 = property on="panel4_7" class="DigNum (strict)"() -> ("Value"=w1003:dbl)  [unwired: 2 in, 2 out]
      n862 = Add(x=w1003, y=w974) -> (x+y=w1002:dbl)
      n863 = Add(x=w1002, y=w975) -> (x+y=w1001:dbl)
      n864 = Add(x=w1001, y=w976) -> (x+y=w1000:dbl)
      n865 = Build Array(w1003, w974, w975, w976, w977, w978, w979, w980, w981, w982, w983, w984, w985, w986) -> (w987:dbl[])
      "Panel 4 array" <- w987
      n866 = Add(x=w1000, y=w977) -> (x+y=w999:dbl)
      n867 = Add(x=w999, y=w978) -> (x+y=w998:dbl)
      n868 = Add(x=w998, y=w979) -> (x+y=w997:dbl)
      n869 = Add(x=w997, y=w980) -> (x+y=w996:dbl)
      n870 = Add(x=w996, y=w981) -> (x+y=w995:dbl)
      n871 = Add(x=w995, y=w982) -> (x+y=w994:dbl)
      n872 = Add(x=w994, y=w983) -> (x+y=w993:dbl)
      n873 = Add(x=w993, y=w984) -> (x+y=w992:dbl)
      n874 = Add(x=w992, y=w985) -> (x+y=w990:dbl)
      n875 = Add(x=w990, y=w986) -> (x+y=w991:dbl)
      n876 = Build Array(w1003, w1002, w1001, w1000, w999, w998, w997, w996, w995, w994, w993, w992, w990, w991) -> (w989:dbl[])
      "Panel 4 acc" <- w989
      n877 = Divide(x=w987, y=1) -> (x/y=w973:dbl[])
    }
    frame #6 {
      # "panel 5"
      n878 = property on="panel5_8" class="DigNum (strict)"() -> ("Value"=w1007:dbl)  [unwired: 2 in, 2 out]
      n879 = property on="panel5_9" class="DigNum (strict)"() -> ("Value"=w1008:dbl)  [unwired: 2 in, 2 out]
      n880 = property on="panel5_10" class="DigNum (strict)"() -> ("Value"=w1009:dbl)  [unwired: 2 in, 2 out]
      n881 = property on="panel5_11" class="DigNum (strict)"() -> ("Value"=w1010:dbl)  [unwired: 2 in, 2 out]
      n882 = property on="panel5_12" class="DigNum (strict)"() -> ("Value"=w1011:dbl)  [unwired: 2 in, 2 out]
      n883 = property on="panel5_13" class="DigNum (strict)"() -> ("Value"=w1012:dbl)  [unwired: 2 in, 2 out]
      n884 = property on="panel5_14" class="DigNum (strict)"() -> ("Value"=w1013:dbl)  [unwired: 2 in, 2 out]
      n885 = property on="panel5_15" class="DigNum (strict)"() -> ("Value"=w1014:dbl)  [unwired: 2 in, 2 out]
      n886 = property on="panel5_16" class="DigNum (strict)"() -> ("Value"=w1015:dbl)  [unwired: 2 in, 2 out]
      n887 = property on="panel5_17" class="DigNum (strict)"() -> ("Value"=w1016:dbl)  [unwired: 2 in, 2 out]
      n888 = property on="panel5_18" class="DigNum (strict)"() -> ("Value"=w1017:dbl)  [unwired: 2 in, 2 out]
      n889 = property on="panel5_19" class="DigNum (strict)"() -> ("Value"=w1018:dbl)  [unwired: 2 in, 2 out]
      n890 = property on="panel5_20" class="DigNum (strict)"() -> ("Value"=w1019:dbl)  [unwired: 2 in, 2 out]
      n891 = property on="panel5_7" class="DigNum (strict)"() -> ("Value"=w1034:dbl)  [unwired: 2 in, 2 out]
      n892 = Add(x=w1034, y=w1007) -> (x+y=w1033:dbl)
      n893 = Add(x=w1033, y=w1008) -> (x+y=w1032:dbl)
      n894 = Add(x=w1032, y=w1009) -> (x+y=w1031:dbl)
      n895 = Build Array(w1034, w1007, w1008, w1009, w1010, w1011, w1012, w1013, w1014, w1015, w1016, w1017, w1018, w1019) -> (w1006:dbl[])
      "Panel 5 array" <- w1006
      n896 = Add(x=w1031, y=w1010) -> (x+y=w1030:dbl)
      n897 = Add(x=w1030, y=w1011) -> (x+y=w1029:dbl)
      n898 = Add(x=w1029, y=w1012) -> (x+y=w1028:dbl)
      n899 = Add(x=w1028, y=w1013) -> (x+y=w1027:dbl)
      n900 = Add(x=w1027, y=w1014) -> (x+y=w1026:dbl)
      n901 = Add(x=w1026, y=w1015) -> (x+y=w1025:dbl)
      n902 = Add(x=w1025, y=w1016) -> (x+y=w1024:dbl)
      n903 = Add(x=w1024, y=w1017) -> (x+y=w1023:dbl)
      n904 = Add(x=w1023, y=w1018) -> (x+y=w1021:dbl)
      n905 = Add(x=w1021, y=w1019) -> (x+y=w1022:dbl)
      n906 = Build Array(w1034, w1033, w1032, w1031, w1030, w1029, w1028, w1027, w1026, w1025, w1024, w1023, w1021, w1022) -> (w1005:dbl[])
      "Panel 5 acc" <- w1005
      n907 = Divide(x=w1006, y=1) -> (x/y=w1004:dbl[])
    }
    frame #7 {
      # "panel 6"
      n908 = property on="panel6_8" class="DigNum (strict)"() -> ("Value"=w1038:dbl)  [unwired: 2 in, 2 out]
      n909 = property on="panel6_9" class="DigNum (strict)"() -> ("Value"=w1039:dbl)  [unwired: 2 in, 2 out]
      n910 = property on="panel6_10" class="DigNum (strict)"() -> ("Value"=w1040:dbl)  [unwired: 2 in, 2 out]
      n911 = property on="panel6_11" class="DigNum (strict)"() -> ("Value"=w1041:dbl)  [unwired: 2 in, 2 out]
      n912 = property on="panel6_12" class="DigNum (strict)"() -> ("Value"=w1042:dbl)  [unwired: 2 in, 2 out]
      n913 = property on="panel6_13" class="DigNum (strict)"() -> ("Value"=w1043:dbl)  [unwired: 2 in, 2 out]
      n914 = property on="panel6_14" class="DigNum (strict)"() -> ("Value"=w1044:dbl)  [unwired: 2 in, 2 out]
      n915 = property on="panel6_15" class="DigNum (strict)"() -> ("Value"=w1045:dbl)  [unwired: 2 in, 2 out]
      n916 = property on="panel6_16" class="DigNum (strict)"() -> ("Value"=w1046:dbl)  [unwired: 2 in, 2 out]
      n917 = property on="panel6_17" class="DigNum (strict)"() -> ("Value"=w1047:dbl)  [unwired: 2 in, 2 out]
      n918 = property on="panel6_18" class="DigNum (strict)"() -> ("Value"=w1048:dbl)  [unwired: 2 in, 2 out]
      n919 = property on="panel6_19" class="DigNum (strict)"() -> ("Value"=w1049:dbl)  [unwired: 2 in, 2 out]
      n920 = property on="panel6_20" class="DigNum (strict)"() -> ("Value"=w1050:dbl)  [unwired: 2 in, 2 out]
      n921 = property on="panel6_7" class="DigNum (strict)"() -> ("Value"=w1065:dbl)  [unwired: 2 in, 2 out]
      n922 = Add(x=w1065, y=w1038) -> (x+y=w1064:dbl)
      n923 = Add(x=w1064, y=w1039) -> (x+y=w1063:dbl)
      n924 = Add(x=w1063, y=w1040) -> (x+y=w1062:dbl)
      n925 = Build Array(w1065, w1038, w1039, w1040, w1041, w1042, w1043, w1044, w1045, w1046, w1047, w1048, w1049, w1050) -> (w1037:dbl[])
      "Panel 6 array" <- w1037
      n926 = Add(x=w1062, y=w1041) -> (x+y=w1061:dbl)
      n927 = Add(x=w1061, y=w1042) -> (x+y=w1060:dbl)
      n928 = Add(x=w1060, y=w1043) -> (x+y=w1059:dbl)
      n929 = Add(x=w1059, y=w1044) -> (x+y=w1058:dbl)
      n930 = Add(x=w1058, y=w1045) -> (x+y=w1057:dbl)
      n931 = Add(x=w1057, y=w1046) -> (x+y=w1056:dbl)
      n932 = Add(x=w1056, y=w1047) -> (x+y=w1055:dbl)
      n933 = Add(x=w1055, y=w1048) -> (x+y=w1054:dbl)
      n934 = Add(x=w1054, y=w1049) -> (x+y=w1052:dbl)
      n935 = Add(x=w1052, y=w1050) -> (x+y=w1053:dbl)
      n936 = Build Array(w1065, w1064, w1063, w1062, w1061, w1060, w1059, w1058, w1057, w1056, w1055, w1054, w1052, w1053) -> (w1036:dbl[])
      "Panel 6 acc" <- w1036
      n937 = Divide(x=w1037, y=1) -> (x/y=w1035:dbl[])
    }
    frame #8 {
      # "panel 7"
      n938 = property on="panel7_8" class="DigNum (strict)"() -> ("Value"=w1069:dbl)  [unwired: 2 in, 2 out]
      n939 = property on="panel7_9" class="DigNum (strict)"() -> ("Value"=w1070:dbl)  [unwired: 2 in, 2 out]
      n940 = property on="panel7_10" class="DigNum (strict)"() -> ("Value"=w1071:dbl)  [unwired: 2 in, 2 out]
      n941 = property on="panel7_11" class="DigNum (strict)"() -> ("Value"=w1072:dbl)  [unwired: 2 in, 2 out]
      n942 = property on="panel7_12" class="DigNum (strict)"() -> ("Value"=w1073:dbl)  [unwired: 2 in, 2 out]
      n943 = property on="panel7_13" class="DigNum (strict)"() -> ("Value"=w1074:dbl)  [unwired: 2 in, 2 out]
      n944 = property on="panel7_14" class="DigNum (strict)"() -> ("Value"=w1075:dbl)  [unwired: 2 in, 2 out]
      n945 = property on="panel7_15" class="DigNum (strict)"() -> ("Value"=w1076:dbl)  [unwired: 2 in, 2 out]
      n946 = property on="panel7_16" class="DigNum (strict)"() -> ("Value"=w1077:dbl)  [unwired: 2 in, 2 out]
      n947 = property on="panel7_17" class="DigNum (strict)"() -> ("Value"=w1078:dbl)  [unwired: 2 in, 2 out]
      n948 = property on="panel7_18" class="DigNum (strict)"() -> ("Value"=w1079:dbl)  [unwired: 2 in, 2 out]
      n949 = property on="panel7_19" class="DigNum (strict)"() -> ("Value"=w1080:dbl)  [unwired: 2 in, 2 out]
      n950 = property on="panel7_20" class="DigNum (strict)"() -> ("Value"=w1081:dbl)  [unwired: 2 in, 2 out]
      n951 = property on="panel7_7" class="DigNum (strict)"() -> ("Value"=w1096:dbl)  [unwired: 2 in, 2 out]
      n952 = Add(x=w1096, y=w1069) -> (x+y=w1095:dbl)
      n953 = Add(x=w1095, y=w1070) -> (x+y=w1094:dbl)
      n954 = Add(x=w1094, y=w1071) -> (x+y=w1093:dbl)
      n955 = Build Array(w1096, w1069, w1070, w1071, w1072, w1073, w1074, w1075, w1076, w1077, w1078, w1079, w1080, w1081) -> (w1068:dbl[])
      "Panel7 array" <- w1068
      n956 = Add(x=w1093, y=w1072) -> (x+y=w1092:dbl)
      n957 = Add(x=w1092, y=w1073) -> (x+y=w1091:dbl)
      n958 = Add(x=w1091, y=w1074) -> (x+y=w1090:dbl)
      n959 = Add(x=w1090, y=w1075) -> (x+y=w1089:dbl)
      n960 = Add(x=w1089, y=w1076) -> (x+y=w1088:dbl)
      n961 = Add(x=w1088, y=w1077) -> (x+y=w1087:dbl)
      n962 = Add(x=w1087, y=w1078) -> (x+y=w1086:dbl)
      n963 = Add(x=w1086, y=w1079) -> (x+y=w1085:dbl)
      n964 = Add(x=w1085, y=w1080) -> (x+y=w1083:dbl)
      n965 = Add(x=w1083, y=w1081) -> (x+y=w1084:dbl)
      n966 = Build Array(w1096, w1095, w1094, w1093, w1092, w1091, w1090, w1089, w1088, w1087, w1086, w1085, w1083, w1084) -> (w1067:dbl[])
      "Panel7 acc" <- w1067
      n967 = Divide(x=w1068, y=1) -> (x/y=w1066:dbl[])
    }
    frame #9 {
      # "radiation2"
      n968 = property on="rad2_7" class="DigNum (strict)"() -> ("Value"=w1111:dbl)  [unwired: 2 in, 2 out]
      n969 = property on="rad2_8" class="DigNum (strict)"() -> ("Value"=w1109:dbl)  [unwired: 2 in, 2 out]
      n970 = property on="rad2_9" class="DigNum (strict)"() -> ("Value"=w1097:dbl)  [unwired: 2 in, 2 out]
      n971 = property on="rad2_10" class="DigNum (strict)"() -> ("Value"=w1098:dbl)  [unwired: 2 in, 2 out]
      n972 = property on="rad2_11" class="DigNum (strict)"() -> ("Value"=w1099:dbl)  [unwired: 2 in, 2 out]
      n973 = property on="rad2_12" class="DigNum (strict)"() -> ("Value"=w1100:dbl)  [unwired: 2 in, 2 out]
      n974 = property on="rad2_13" class="DigNum (strict)"() -> ("Value"=w1101:dbl)  [unwired: 2 in, 2 out]
      n975 = property on="rad2_14" class="DigNum (strict)"() -> ("Value"=w1102:dbl)  [unwired: 2 in, 2 out]
      n976 = property on="rad2_15" class="DigNum (strict)"() -> ("Value"=w1103:dbl)  [unwired: 2 in, 2 out]
      n977 = property on="rad2_16" class="DigNum (strict)"() -> ("Value"=w1104:dbl)  [unwired: 2 in, 2 out]
      n978 = property on="rad2_17" class="DigNum (strict)"() -> ("Value"=w1105:dbl)  [unwired: 2 in, 2 out]
      n979 = property on="rad2_18" class="DigNum (strict)"() -> ("Value"=w1106:dbl)  [unwired: 2 in, 2 out]
      n980 = property on="rad2_19" class="DigNum (strict)"() -> ("Value"=w1107:dbl)  [unwired: 2 in, 2 out]
      n981 = property on="rad2_20" class="DigNum (strict)"() -> ("Value"=w1108:dbl)  [unwired: 2 in, 2 out]
      n982 = Build Array(w1111, w1109, w1097, w1098, w1099, w1100, w1101, w1102, w1103, w1104, w1105, w1106, w1107, w1108) -> (→"radiation_array 2":dbl[])
    }
    frame #10 {
      # "radiation3"
      n983 = property on="rad1_7" class="DigNum (strict)"() -> ("Value"=w1126:dbl)  [unwired: 2 in, 2 out]
      n984 = property on="rad1_8" class="DigNum (strict)"() -> ("Value"=w1124:dbl)  [unwired: 2 in, 2 out]
      n985 = property on="rad1_9" class="DigNum (strict)"() -> ("Value"=w1112:dbl)  [unwired: 2 in, 2 out]
      n986 = property on="rad1_10" class="DigNum (strict)"() -> ("Value"=w1113:dbl)  [unwired: 2 in, 2 out]
      n987 = property on="rad1_11" class="DigNum (strict)"() -> ("Value"=w1114:dbl)  [unwired: 2 in, 2 out]
      n988 = property on="rad1_12" class="DigNum (strict)"() -> ("Value"=w1115:dbl)  [unwired: 2 in, 2 out]
      n989 = property on="rad1_13" class="DigNum (strict)"() -> ("Value"=w1116:dbl)  [unwired: 2 in, 2 out]
      n990 = property on="rad1_14" class="DigNum (strict)"() -> ("Value"=w1117:dbl)  [unwired: 2 in, 2 out]
      n991 = property on="rad1_15" class="DigNum (strict)"() -> ("Value"=w1118:dbl)  [unwired: 2 in, 2 out]
      n992 = property on="rad1_16" class="DigNum (strict)"() -> ("Value"=w1119:dbl)  [unwired: 2 in, 2 out]
      n993 = property on="rad1_17" class="DigNum (strict)"() -> ("Value"=w1120:dbl)  [unwired: 2 in, 2 out]
      n994 = property on="rad1_18" class="DigNum (strict)"() -> ("Value"=w1121:dbl)  [unwired: 2 in, 2 out]
      n995 = property on="rad1_19" class="DigNum (strict)"() -> ("Value"=w1122:dbl)  [unwired: 2 in, 2 out]
      n996 = property on="rad1_20" class="DigNum (strict)"() -> ("Value"=w1123:dbl)  [unwired: 2 in, 2 out]
      n997 = Build Array(w1126, w1124, w1112, w1113, w1114, w1115, w1116, w1117, w1118, w1119, w1120, w1121, w1122, w1123) -> (→"radiation_array 3":dbl[])
    }
    frame #11 {
      n998 = property on="Panel 5 array" class="Arr (strict)"() -> ("Value"=w1140:dbl[])  [unwired: 2 in, 2 out]
      n999 = property on="Panel 4 array" class="Arr (strict)"() -> ("Value"=w1139:dbl[])  [unwired: 2 in, 2 out]
      n1000 = property on="Panel7 array" class="Arr (strict)"() -> ("Value"=w1142:dbl[])  [unwired: 2 in, 2 out]
      n1001 = property on="Panel 1 array" class="Arr (strict)"() -> ("Value"=w1136:dbl[])  [unwired: 2 in, 2 out]
      n1002 = property on="Panel 2 array" class="Arr (strict)"() -> ("Value"=w1137:dbl[])  [unwired: 2 in, 2 out]
      n1003 = property on="Panel 3 array" class="Arr (strict)"() -> ("Value"=w1138:dbl[])  [unwired: 2 in, 2 out]
      n1004 = property on="Panel 6 array" class="Arr (strict)"() -> ("Value"=w1141:dbl[])  [unwired: 2 in, 2 out]
      n1005 = property on="Panel 1 acc" class="Arr (strict)"() -> ("Value"=w1129:dbl[])  [unwired: 2 in, 2 out]
      n1006 = property on="Panel 2_acc" class="Arr (strict)"() -> ("Value"=w1130:dbl[])  [unwired: 2 in, 2 out]
      n1007 = property on="Panel 3 acc" class="Arr (strict)"() -> ("Value"=w1131:dbl[])  [unwired: 2 in, 2 out]
      n1008 = property on="Panel 4 acc" class="Arr (strict)"() -> ("Value"=w1132:dbl[])  [unwired: 2 in, 2 out]
      n1009 = property on="Panel 5 acc" class="Arr (strict)"() -> ("Value"=w1133:dbl[])  [unwired: 2 in, 2 out]
      n1010 = property on="Panel 6 acc" class="Arr (strict)"() -> ("Value"=w1134:dbl[])  [unwired: 2 in, 2 out]
      n1011 = property on="Panel7 acc" class="Arr (strict)"() -> ("Value"=w1135:dbl[])  [unwired: 2 in, 2 out]
      n1012 = Divide(x=w1136, y=0.04) -> (x/y=w1150:dbl[])
      n1013 = Divide(x=w1137, y=0.123) -> (x/y=w1151:dbl[])
      n1014 = Divide(x=w1138, y=2) -> (x/y=w1152:dbl[])
      n1015 = Divide(x=w1139, y=50) -> (x/y=w1153:dbl[])
      n1016 = Divide(x=w1140, y=50) -> (x/y=w1154:dbl[])
      n1017 = Divide(x=w1141, y=30) -> (x/y=w1155:dbl[])
      n1018 = Divide(x=w1142, y=30) -> (x/y=w1156:dbl[])
      n1019 = property on="radiation_array" class="Arr (strict)"() -> ("Value"=w1157:dbl[])  [unwired: 2 in, 2 out]
      n1020 = property on="radiation_array 2" class="Arr (strict)"() -> ("Value"=w1158:dbl[])  [unwired: 2 in, 2 out]
      n1021 = property on="radiation_array 3" class="Arr (strict)"() -> ("Value"=w1128:dbl[])  [unwired: 2 in, 2 out]
      n1022 = Build Array(w1136, w1137, w1138, w1139, w1140, w1141, w1142, w1129, w1130, w1131, w1132, w1133, w1134, w1135, w1150, w1151, w1152, w1153, w1154, w1155, w1156, w1157, w1158, w1128) -> (w1127:dbl[][])
    }
  }
  n1023 = Add Array Elements(numeric array=w9) -> (sum=w65:dbl)
  n1024 = Divide(x=w65, y=14.0) -> (x/y=w51:dbl)
  n1025 = Add Array Elements(numeric array=w61) -> (sum=w63:dbl)
  n1026 = Divide(x=w63, y=14.0) -> (x/y=w50:dbl)
  n1027 = Add Array Elements(numeric array=w44) -> (sum=w46:dbl)
  n1028 = Divide(x=w46, y=14.0) -> (x/y=w35:dbl)
  n1029 = Add Array Elements(numeric array=w58) -> (sum=w60:dbl)
  n1030 = Divide(x=w60, y=14.0) -> (x/y=w49:dbl)
  n1031 = Add Array Elements(numeric array=w41) -> (sum=w43:dbl)
  n1032 = Divide(x=w43, y=14.0) -> (x/y=w34:dbl)
  n1033 = Add Array Elements(numeric array=w55) -> (sum=w57:dbl)
  n1034 = Divide(x=w57, y=14.0) -> (x/y=w48:dbl)
  n1035 = Add Array Elements(numeric array=w38) -> (sum=w40:dbl)
  n1036 = Divide(x=w40, y=14.0) -> (x/y=w33:dbl)
  n1037 = Number To Fractional String(number=w2, precision (6)=i16 3) -> (F-format string=w7:string[][])  [unwired: 2 in]
  n1038 = Add Array Elements(numeric array=w52) -> (sum=w54:dbl)
  n1039 = Add Array Elements(numeric array=w10) -> (sum=w37:dbl)
  n1040 = Divide(x=w54, y=14.0) -> (x/y=w47:dbl)
  n1041 = Divide(x=w37, y=14.0) -> (x/y=w32:dbl)
  n1042 = Build Array(w35, w34, w33, w32) -> (w30:dbl[])
  n1043 = Build Array(w51, w50, w49, w48, w47) -> (w31:dbl[])
  n1044 = Build Array (concatenate)("column headers", w7) -> (w5:string[][])
  n1045 = Number To Fractional String(number=w31, precision (6)=w22) -> (F-format string=w29:string[])  [unwired: 2 in]
  n1046 = Number To Fractional String(number=w30, precision (6)=w22) -> (F-format string=w27:string[])  [unwired: 2 in]
  n1047 = Insert Into Array(array=w5, index (col)=0 ("disabled index (col)"), new element=w4) -> (w1:string[][])  [unwired: 1 in]
  "output array 4" <- w1
  n1048 = property on="file path (dialog if empty)" class="Path"() -> ("Value"=w16:path)  [unwired: 2 in, 2 out]
  n1049 = Build Array(w9, w61, w58, w55, w52, w69, w68, w67, w66, w44, w41, w38, w10) -> (w26:dbl[][])
  "appended array" <- w26
  n1050 = Insert Into Array(array=w29, new element #1=w28, new element #2=w28, new element #3=w28, new element #4=w28, new element #5=w27) -> (w23:string[])  [unwired: 1 in]
  "output array" <- w23
  n1051 = Strip Path(path=w16) -> (stripped path=w15:path, name=w13:string)
  n1052 = Path To String(path=w15) -> (string=w17:string)
  n1053 = Concatenate Strings(w17, "\\report_" ("string"), w13) -> (w12:string)
  n1054 = Number To Fractional String(number=w26, precision (6)=w22) -> (F-format string=w25:string[][])  [unwired: 2 in]
  n1055 = String To Path(string=w12) -> (path=w11:path)
  n1056 = call-poly <vilib>:"Write To Spreadsheet File.vi"("2D data"=w1, "file path (dialog if empty)"=w11) -> ()  [unwired: 6 in, 1 out]
  n1057 = Insert Into Array(array=w25, index (col)=14 ("disabled index (col)"), new element=w23) -> (w21:string[][])  [unwired: 1 in]
  "output array 3" <- w21
  n1058 = Build Array (concatenate)("column headers", w21) -> (w20:string[][])
  n1059 = Insert Into Array(array=w20, index (col)=0 ("disabled index (col)"), new element=w4) -> (→"output array 2":string[][])  [unwired: 1 in]
